vi "Edit a Button--Material.vi"() -> ()   [LabVIEW 2021, in "TSC Button Editor.lvclass"]
doc: "Edit/create buttons based on a few built-in templates.\n\n<b>Code Developed By:</b>\nTechnology Service Corporation\nwww.tsc.com/atcs\n\nDeveloper:\nDaniel Coons"
uses:
  _button-editor/TSC Button Editor.lvclass
  _button-editor/TSC Button Editor.lvclass/TSC Button Editor.ctl
  <vilib>/Utility/miscctls.llb/LVPositionTypeDef.ctl
  _button-editor/Image List Column--constant.vi
  _button-editor/Button Editor Config--constant.vi
  controls/subpanel--button preview.vi
  <vilib>/Utility/libraryn.llb/Get File Extension.vi
  <vilib>/Utility/colorconv.llb/RGB to Color.vi
  <vilib>/Utility/file.llb/Dflt Data Dir.vi
  <vilib>/Utility/libraryn.llb/Check if File or Folder Exists.vi
  <vilib>/Utility/libraryn.llb/Create Directory Recursive.vi
  user32.dll
  Material Theme/Material Theme.lvclass
  Material-Scheme/Material-Scheme.lvclass
panel:
  in  "Save For:":string(combo)
  in  "Tab Control 2":enum32{"Button Format", "Glyphs"}(tab)
  in  "Lock Text in Center?":bool
  in  "update text format":bool
  in  "Boolean Colors":T1={"false color"={"border"=15922170, "fill"=15922170}, "true color"={"border"=14936305, "fill"=14936305}, "click false color"={"border"=14410221, "fill"=14410221}, "click true color"={"border"=14410221, "fill"=14410221}, "hover false color"={"border"=14540516, "fill"=14540516}, "hover true color"={"border"=14540516, "fill"=14540516}}
  in  "Boolean Text Format":T2={"Font:Color"=3563918, "Font:Bold?"=TRUE, "Font:Name"="App Font", "Font:Size"=22}
  in  "Boolean Text":string
  in  "update colors":bool
  in  "Button Size":cluster{"Width":u32, "Height":u32}={"Width"=204, "Height"=48}
  in  "update button size":bool
  in  "Button Text Location":cluster{"Left":i32, "Top":i32}
  in  "update button text location":bool
  in  "edit":bool
  out "Images":T3(array[cluster]) caption="Array"
  in  "Filter":string
  out "images directory":path
  in  "Button Family":u16(ring) items=["(1) Small Button Single Image 24px", "(2) Small Button Text Only", "(3) Large Button Single Image 40px", "(4) Large Button Text Only", "(5) Small Button Multi Image 24px", "(6) Large Button Multi Image 40px", "(7) Floating Action Button (FAB)"]
  in  "Color Level":u16(ring) items=["Primary", "Secondary", "Tertiary", "Error", "Primary Fixed", "Secondary Fixed", "Tertiary Fixed"]
  in  "Theme":u16(ring) items=["Light Theme", "Light Medium Contrast", "Light High Contrast", "Dark Theme", "Dark Medium Contrast", "Dark High Constrast"]
  in  "theme path":path
  in  "Open":bool
  in  "Button Type":u16(ring) items=["elevated--rectangular--icon.ctl", "elevated--rounded--icon.ctl", "filled--rectangular--icon.ctl", "filled--rounded--icon.ctl", "nooutline--rectangular--icon.ctl", "nooutline--rounded--icon.ctl", "outline--rectangular--icon.ctl", "outline--rounded--icon.ctl", "tonal--rectangular--icon.ctl", "tonal--rounded--icon.ctl", "transparent--rectangular--icon.ctl", "transparent--rounded--icon.ctl"]
  in  "Tab Control":enum32{"Button Formatting"}(tab)
  in  "Image Color":u32(colorbox)=3563918
  in  "Button Image":path
  in  "Button Images":T4
  in  "Multiple Colors":T5={"False Color"=3563918, "True Color"=3563918, "True Press"=3563918, "False Press"=3563918}
  out "b":u8
  out "g":u8
  out "r":u8
  out "Color":u32(colorbox)
  in  "Hex Color":u32 max=16777215 format="%06x"
  in  "close":bool
  out "header":bool
  in  "Save":bool
  out "error out":errorcluster
  # "Download a folder of icons here: https://github.com/danielcoons/material-icons-toolkit<Material-Toolkit> to easily sort by size and connect to directory"
  # "drag and drop on glyph Button Image path control to add"
  # "Note: match the size of the replacement image so scaling is correct.\nNormal size: 24x24px, Large size: 40x40px, Icon size: 30x30px\n\nFor other desired sizes, save the control and open it in LabVIEW. Use the edit mode features to replace the picture items. Making sure the image doesn't try to resize is important for it to look correct."
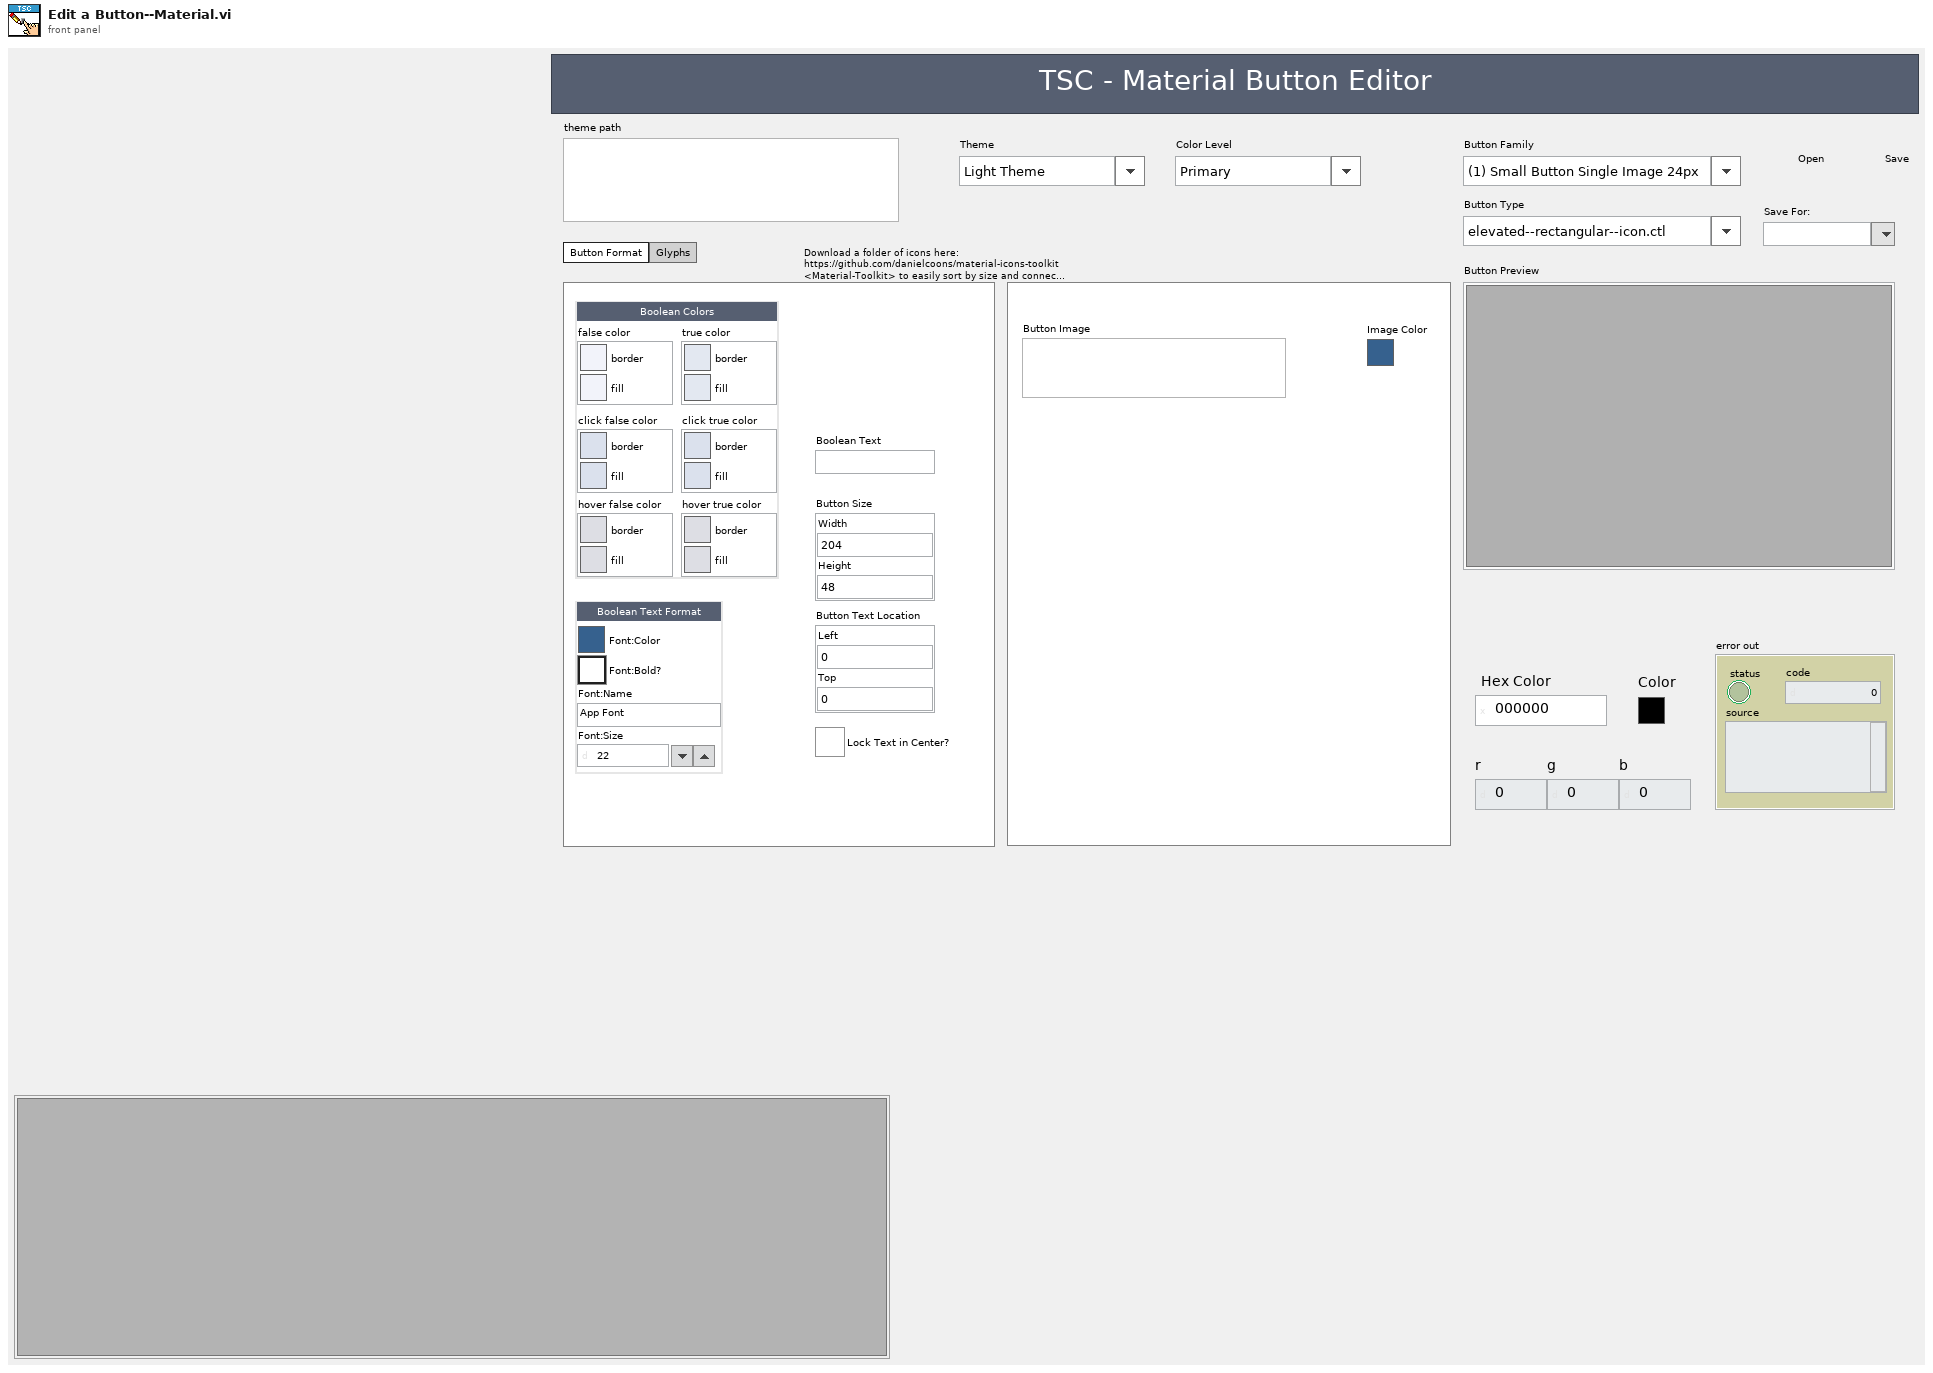
[diagram p1: front panel]
types:
  T1 = cluster{"false color":cluster{"border":u32, "fill":u32}, "true color":cluster{"border":u32, "fill":u32}, "click false color":cluster{"border":u32, "fill":u32}, "click true color":cluster{"border":u32, "fill":u32}, "hover false color":cluster{"border":u32, "fill":u32}, "hover true color":cluster{"border":u32, "fill":u32}}
  T2 = cluster{"Font:Color":u32, "Font:Bold?":bool, "Font:Name":string, "Font:Size":u32}
  T3 = cluster{"2D Picture":picture, "path":path, "image-name":string}[][]
  T4 = cluster{"False Image":path, "True Image":path, "True Press":path, "False Press":path}
  T5 = cluster{"False Color":u32, "True Color":u32, "True Press":u32, "False Press":u32}
  T6 = cluster{"2D Picture":picture, "path":path, "image-name":string}[]
  T7 = typedef "TSC Button Editor.lvclass/User Events--typedef.ctl" = cluster{"update colors":refnum<user-event>, "update boolean data":refnum<user-event>, "update image":refnum<user-event>, "update multi image":refnum<user-event>}
  T8 = typedef "LVPositionTypeDef.ctl" = cluster{"Left":i32, "Top":i32}
  T9 = enum32{"invalid VI type", "Standard VI", "Control VI", "Global VI", "Polymorphic VI", "Configuration VI", "SubSystem", "Facade VI", "Method VI", "Statechart Diagram VI"}
  T10 = typedef "LVBoundsTypeDef.ctl" = cluster{"Width":u32, "Height":u32}
  T11 = cluster{"2D Picture":picture, "path":path, "image-name":string}
  T12 = typedef "LVPoint32TypeDef.ctl" = cluster{"Horizontal":i32, "Vertical":i32}
  T13 = cluster{"data name":string, "drag data":variant}[]
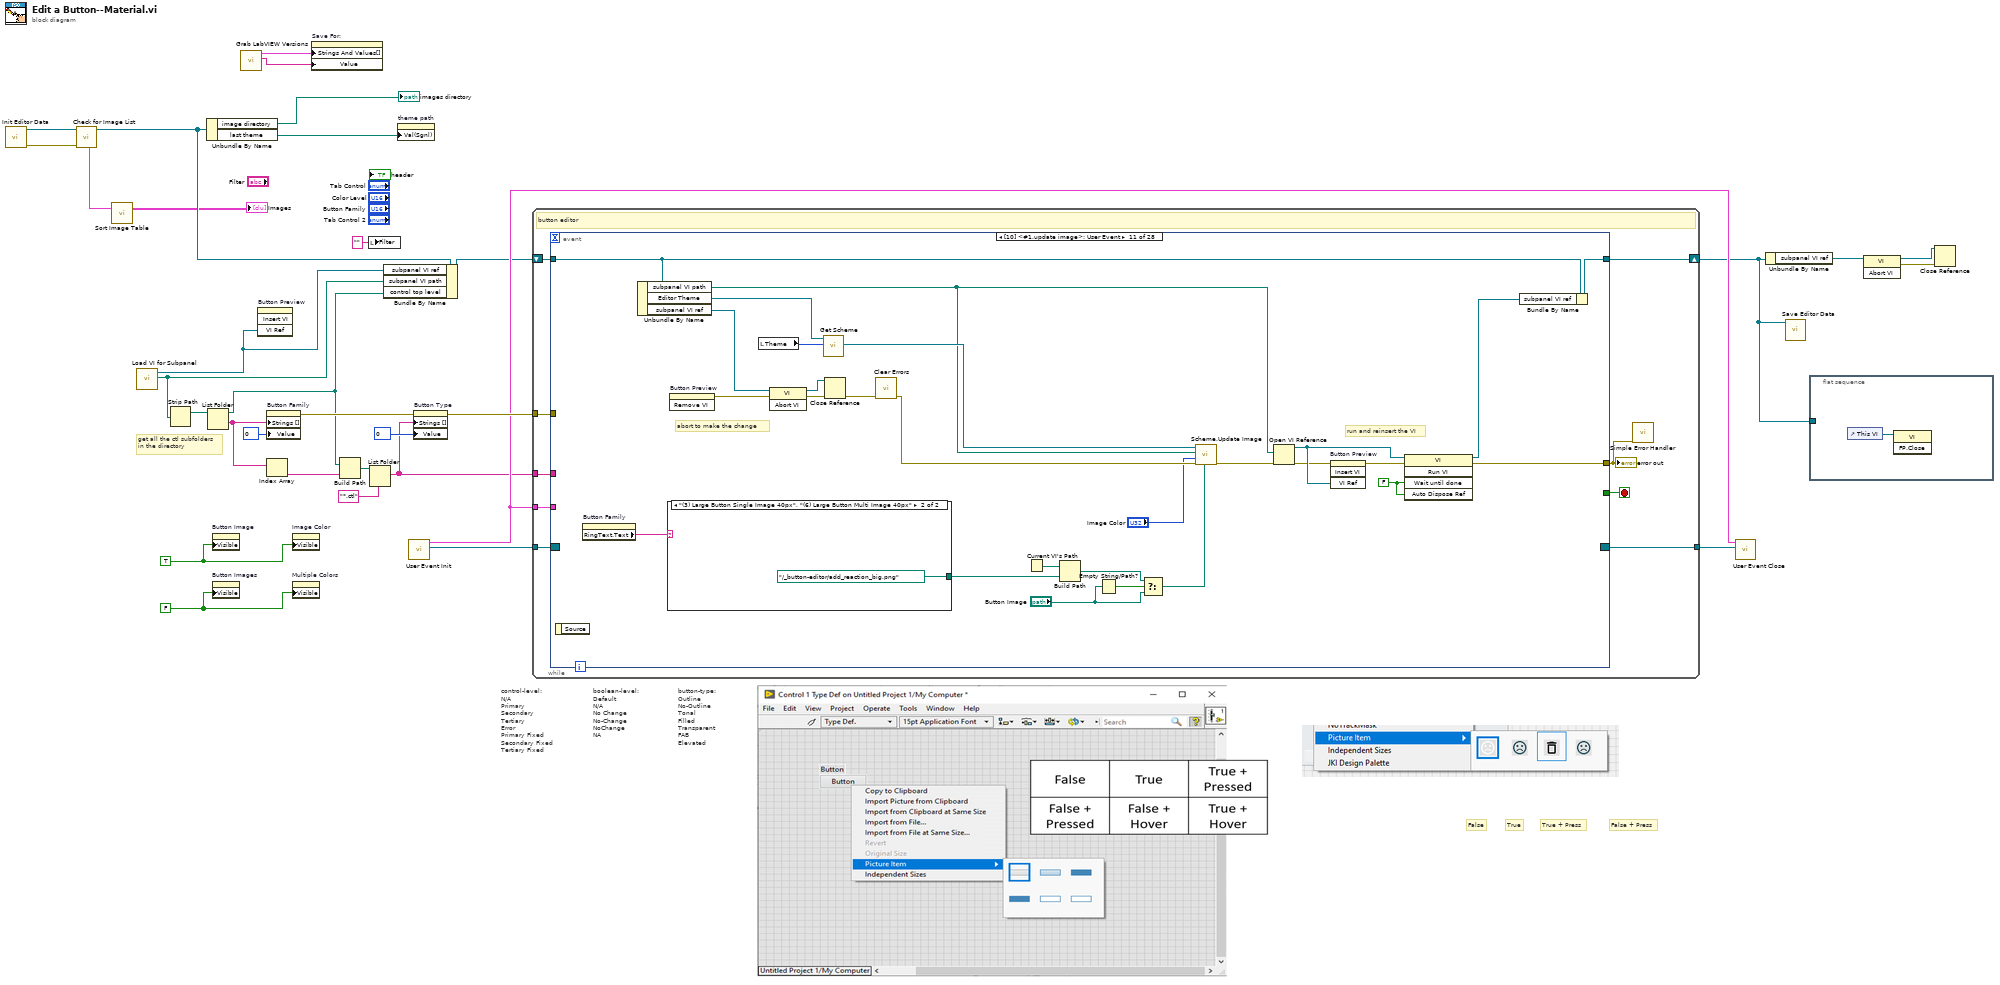
[diagram p0: block diagram]
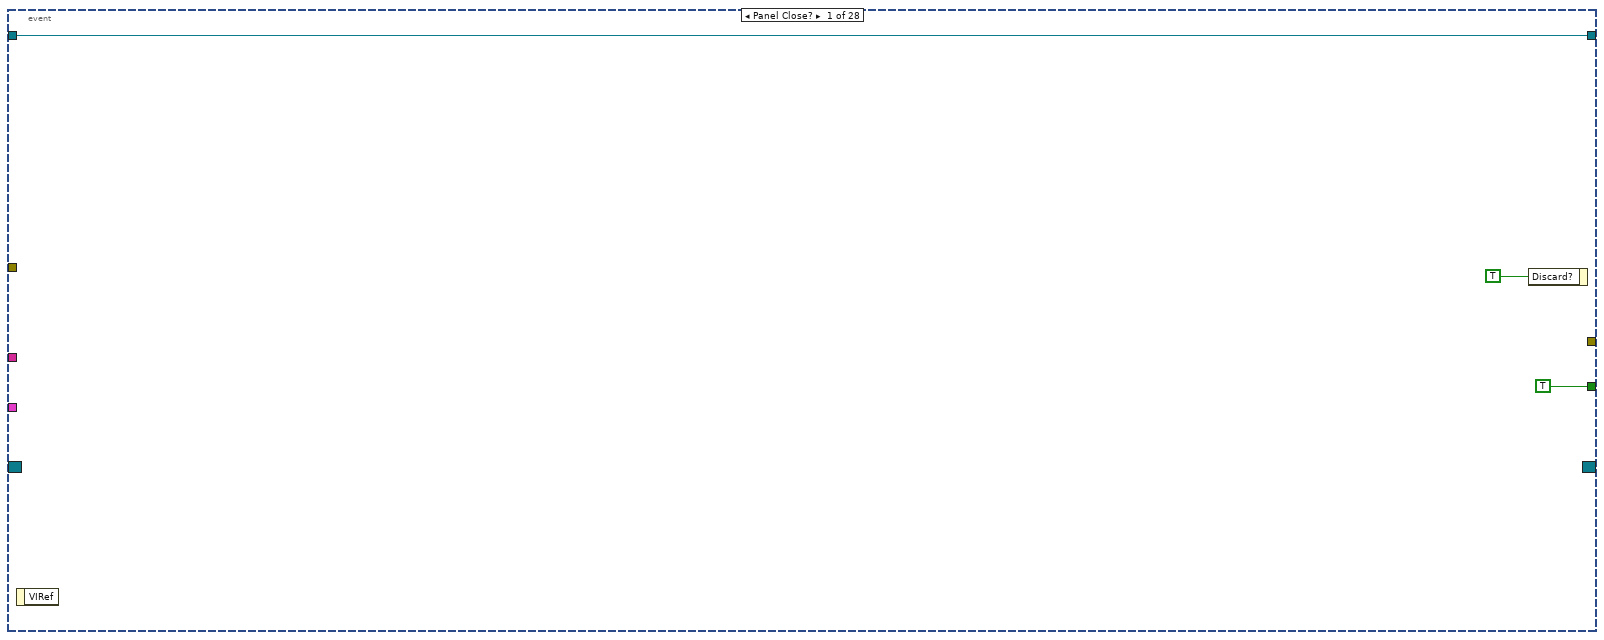
[diagram p2: hidden frame]
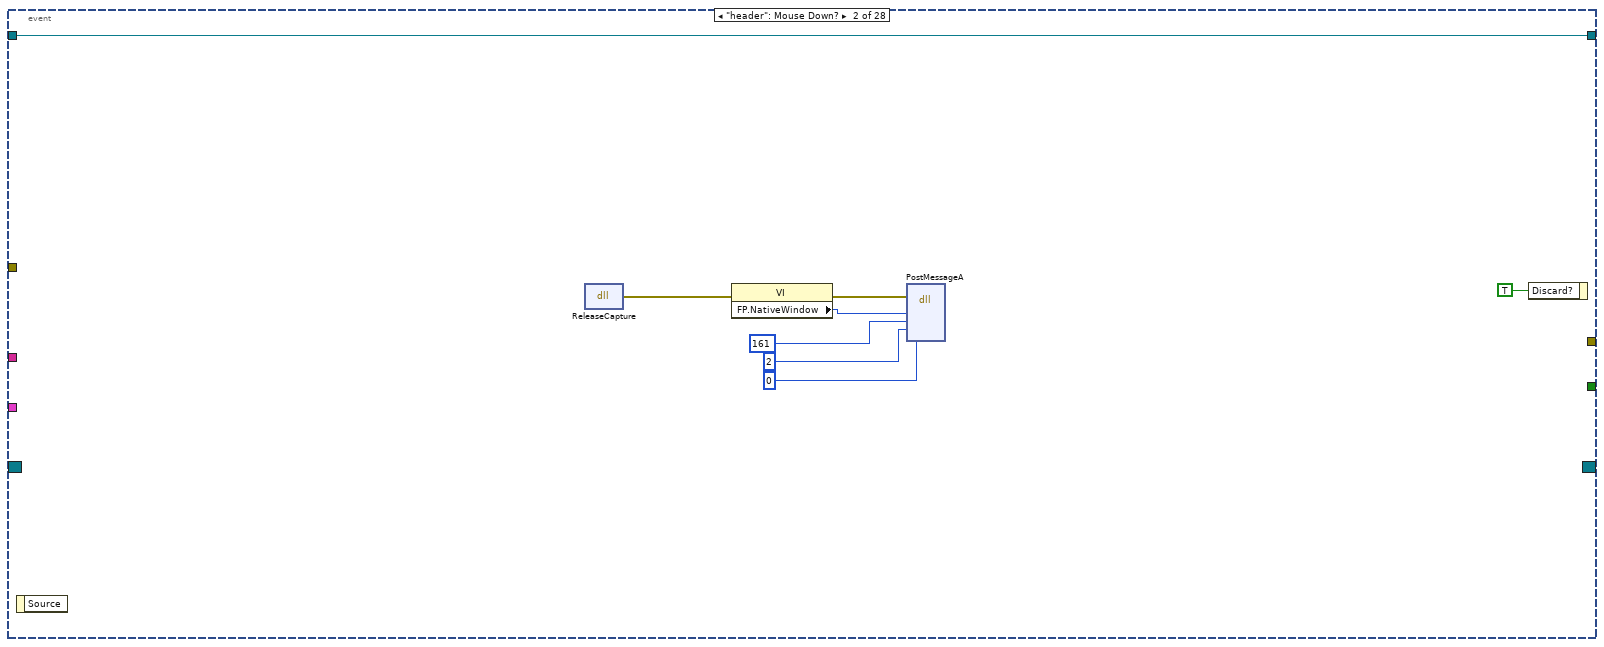
[diagram p3: hidden frame]
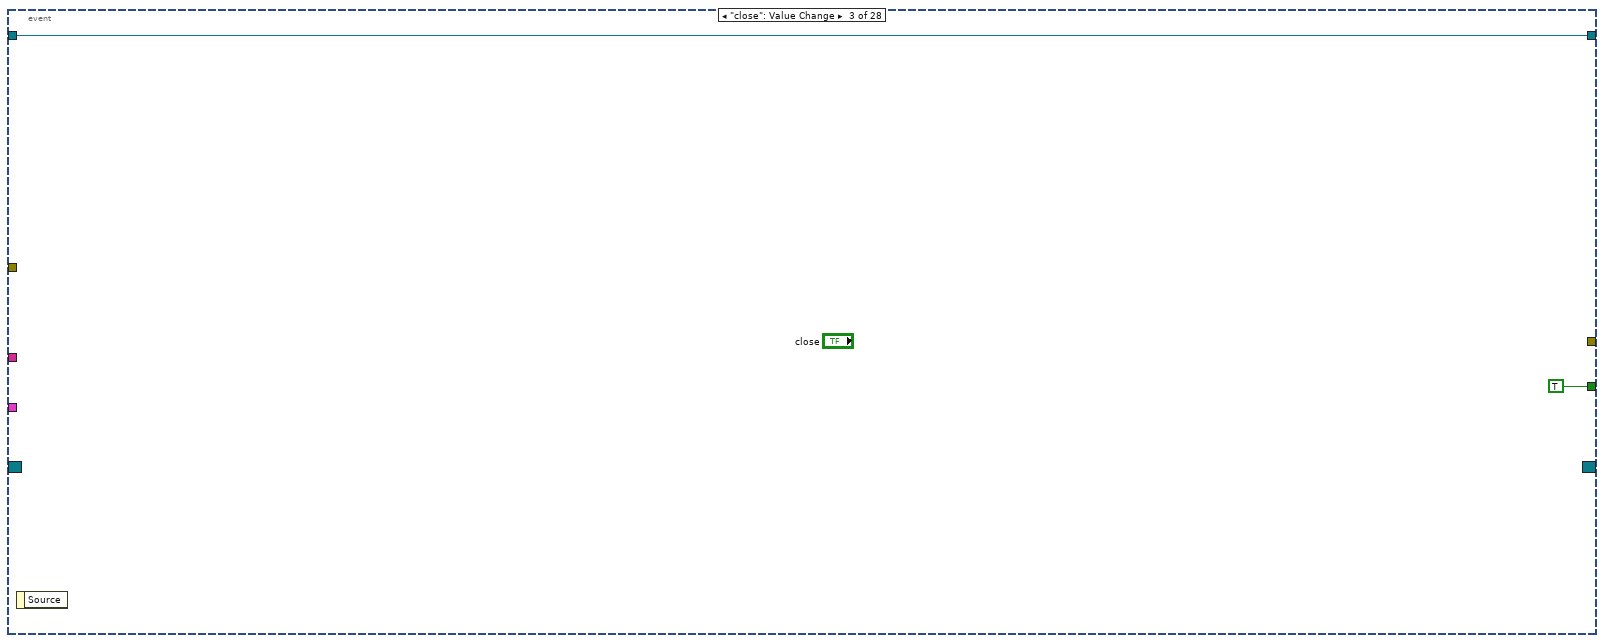
[diagram p4: hidden frame]
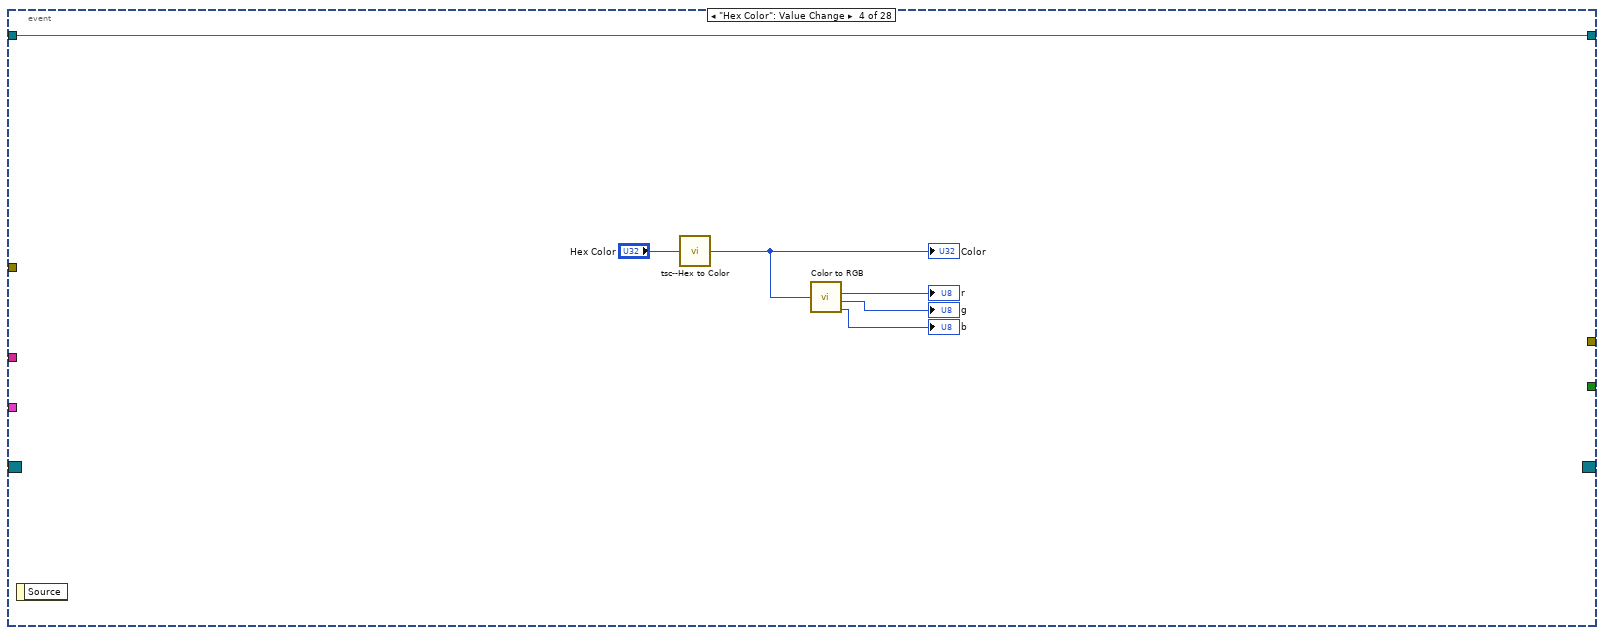
[diagram p5: hidden frame]
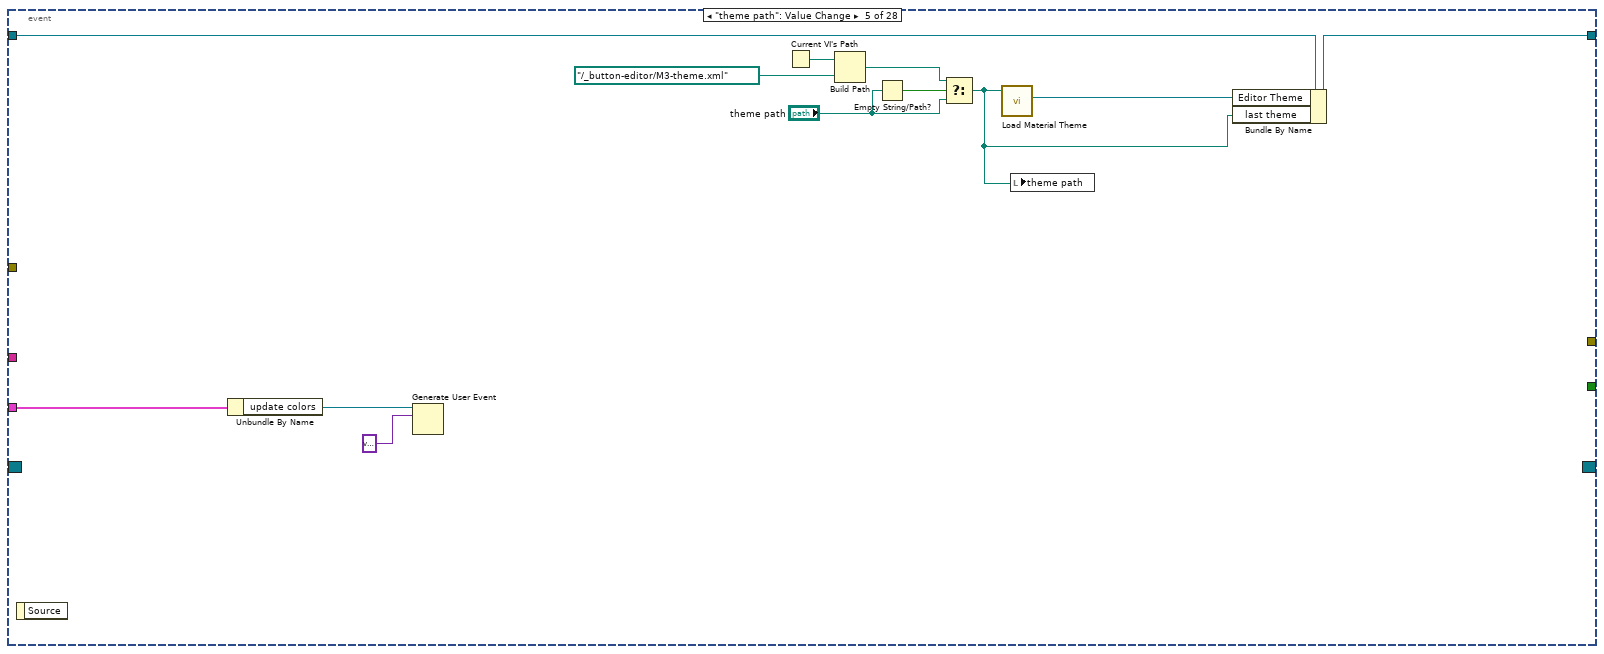
[diagram p6: hidden frame]
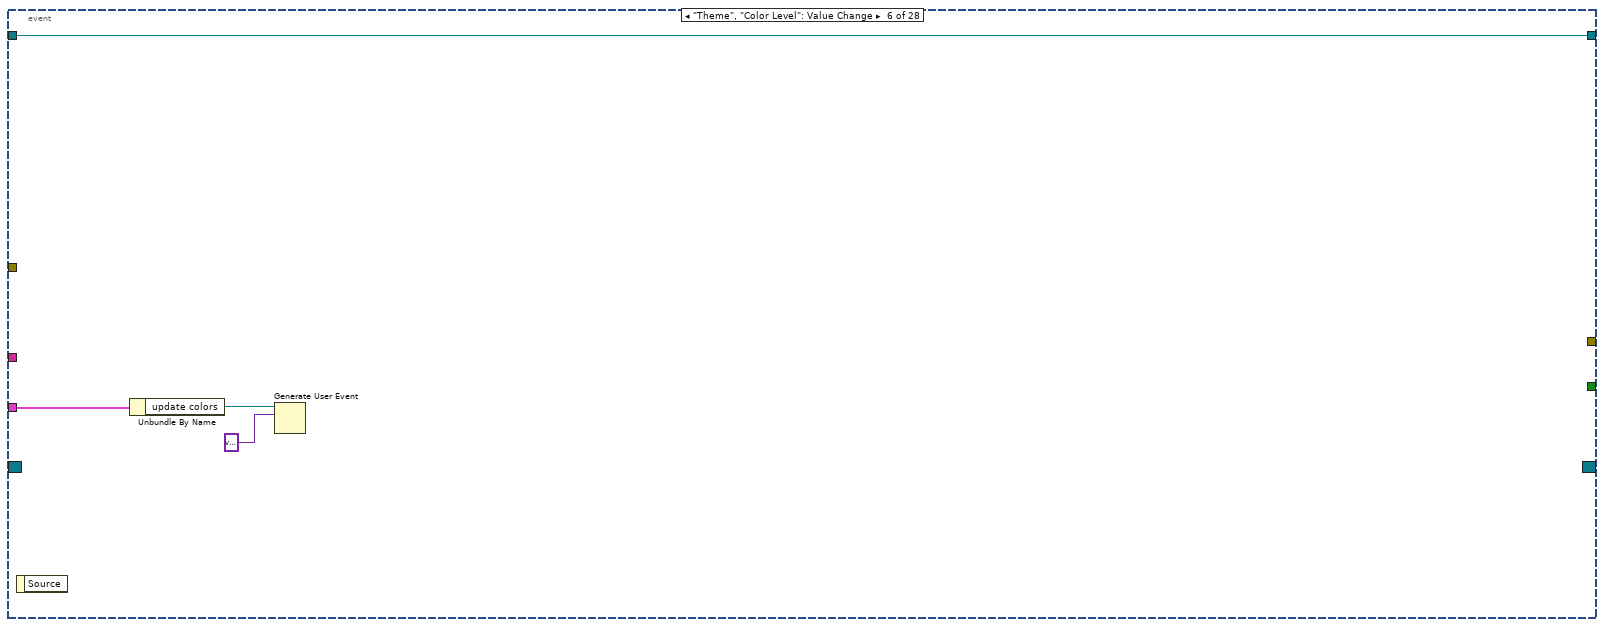
[diagram p7: hidden frame]
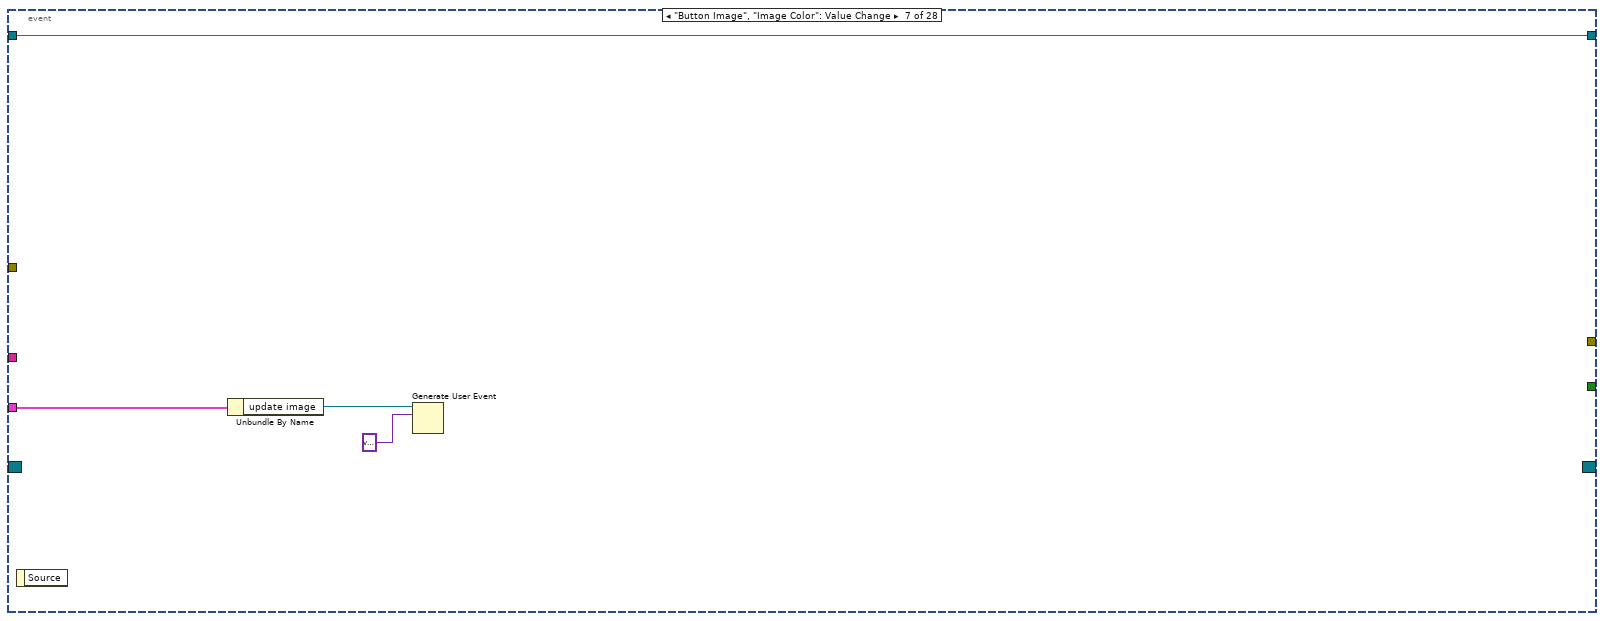
[diagram p8: hidden frame]
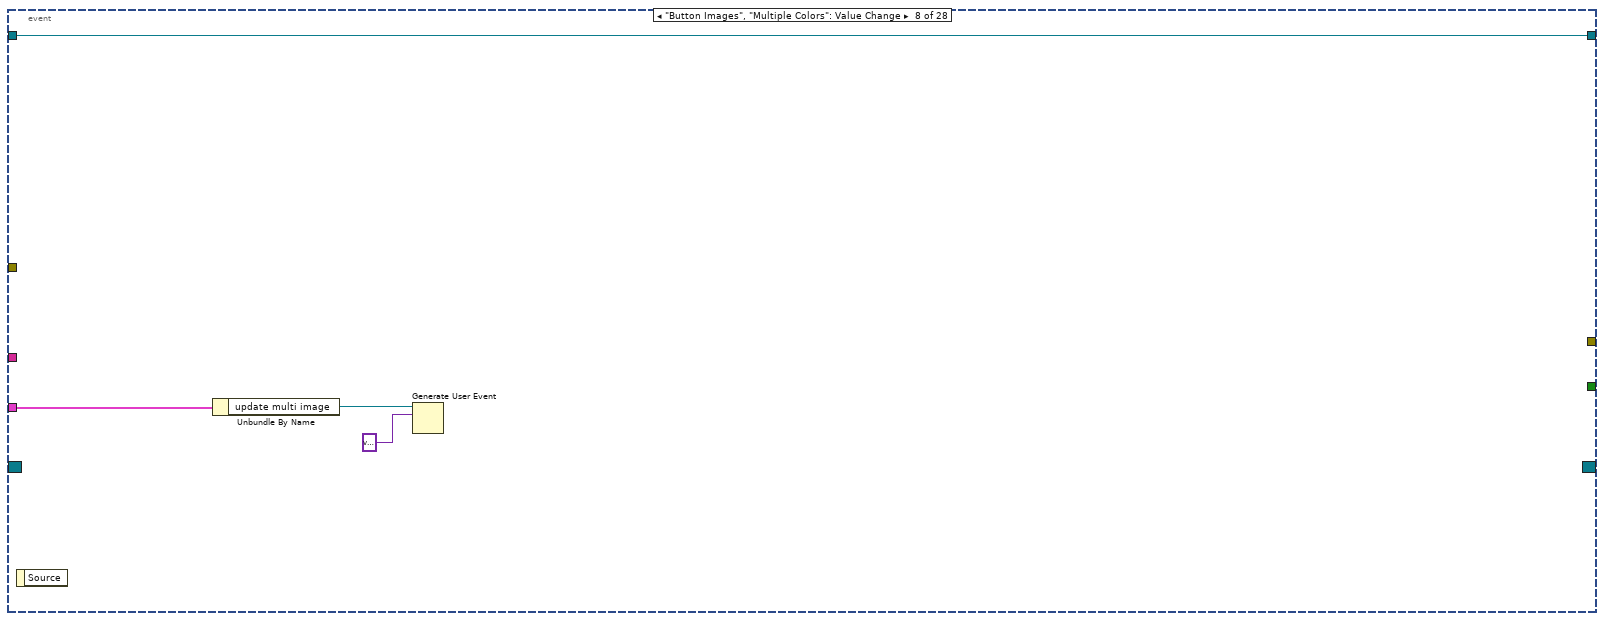
[diagram p9: hidden frame]
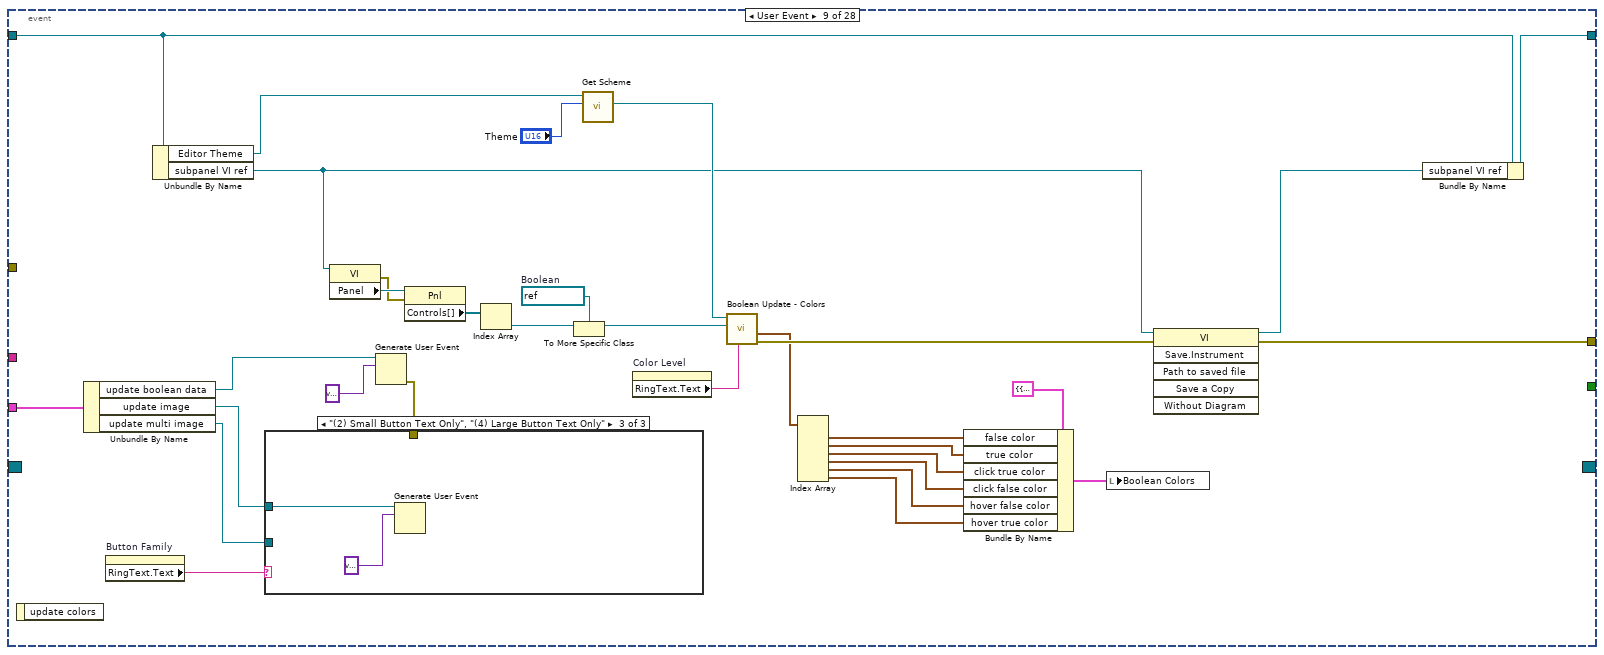
[diagram p10: hidden frame]
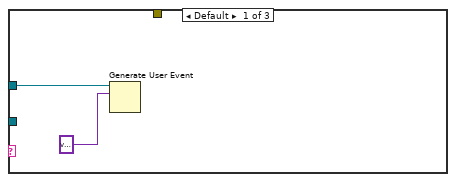
[diagram p11: hidden frame]
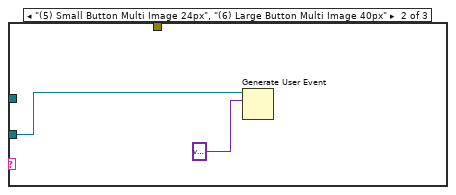
[diagram p12: hidden frame]
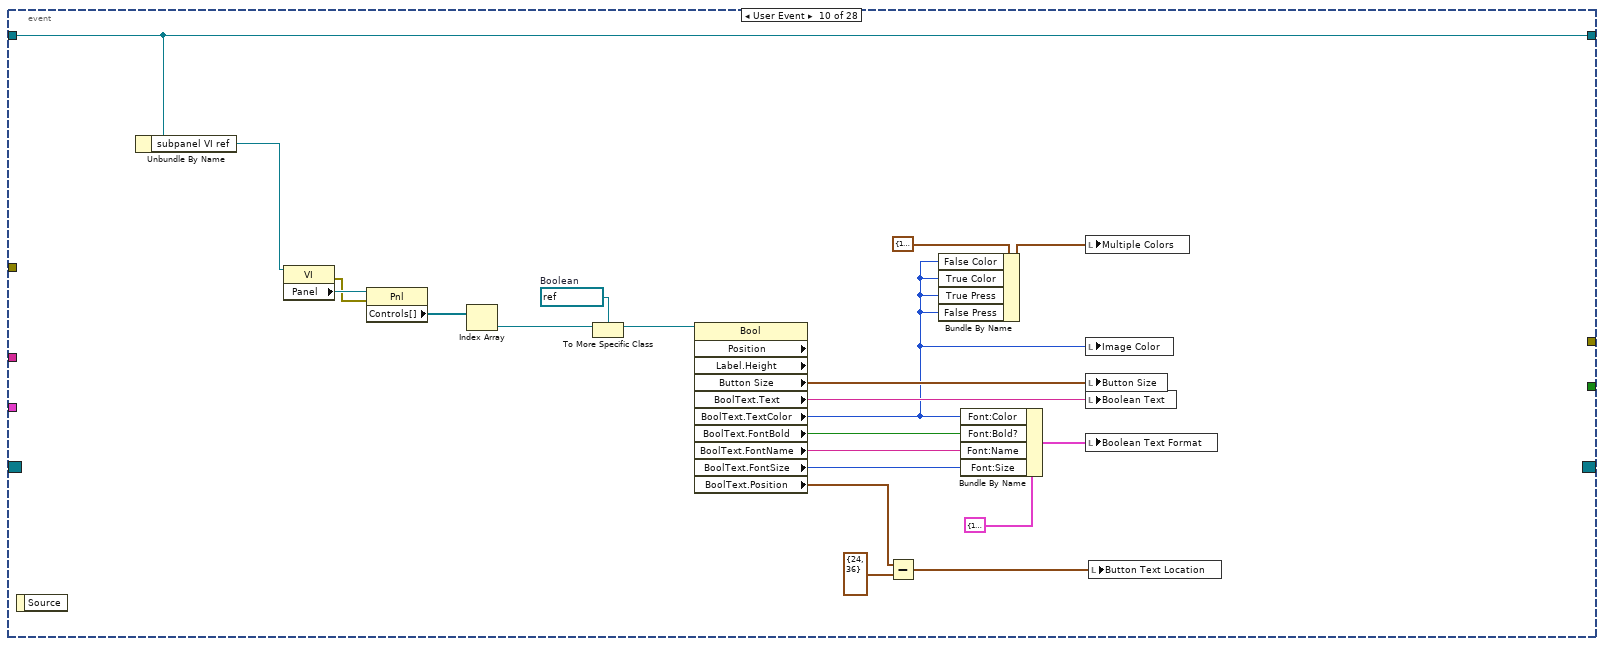
[diagram p13: hidden frame]
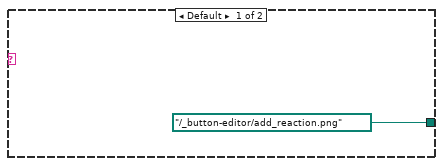
[diagram p14: hidden frame]
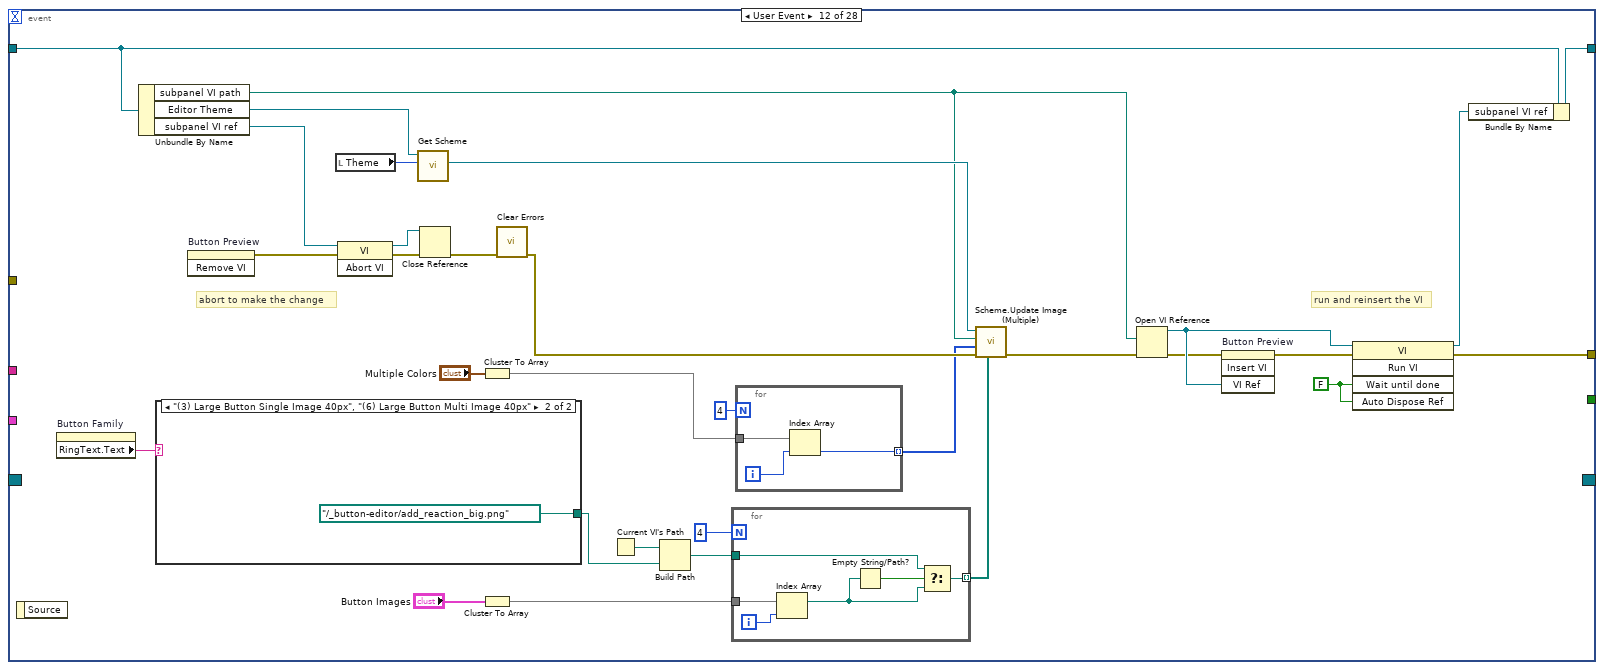
[diagram p15: hidden frame]
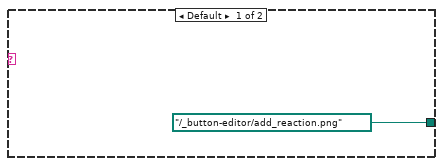
[diagram p16: hidden frame]
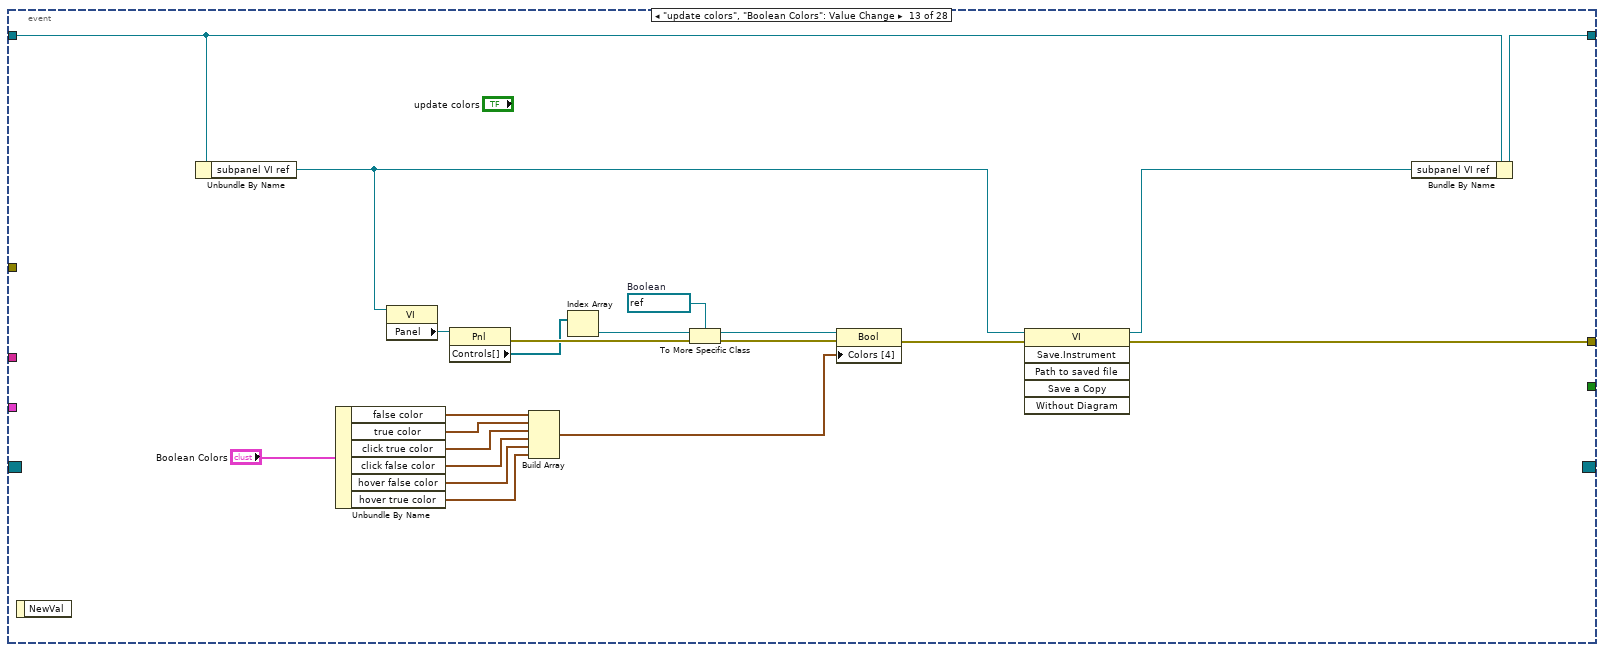
[diagram p17: hidden frame]
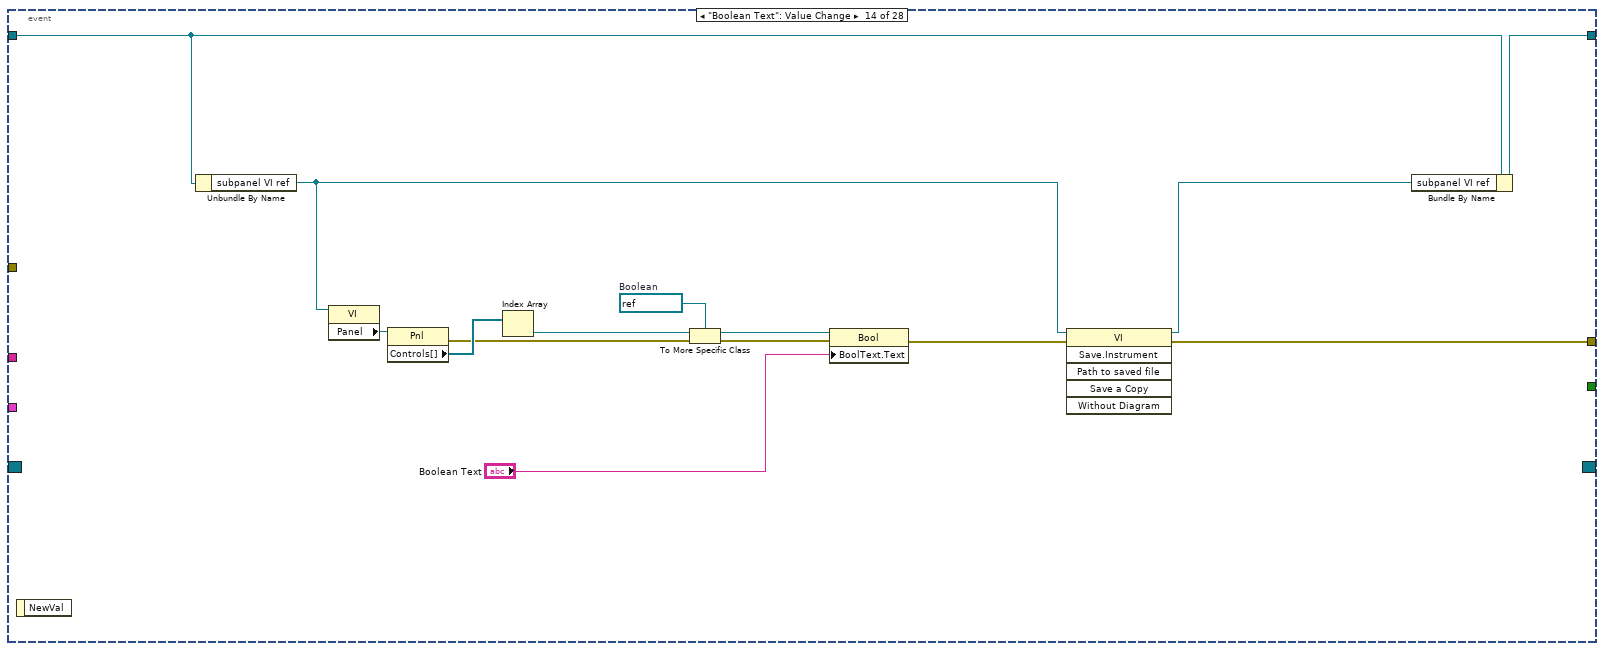
[diagram p18: hidden frame]
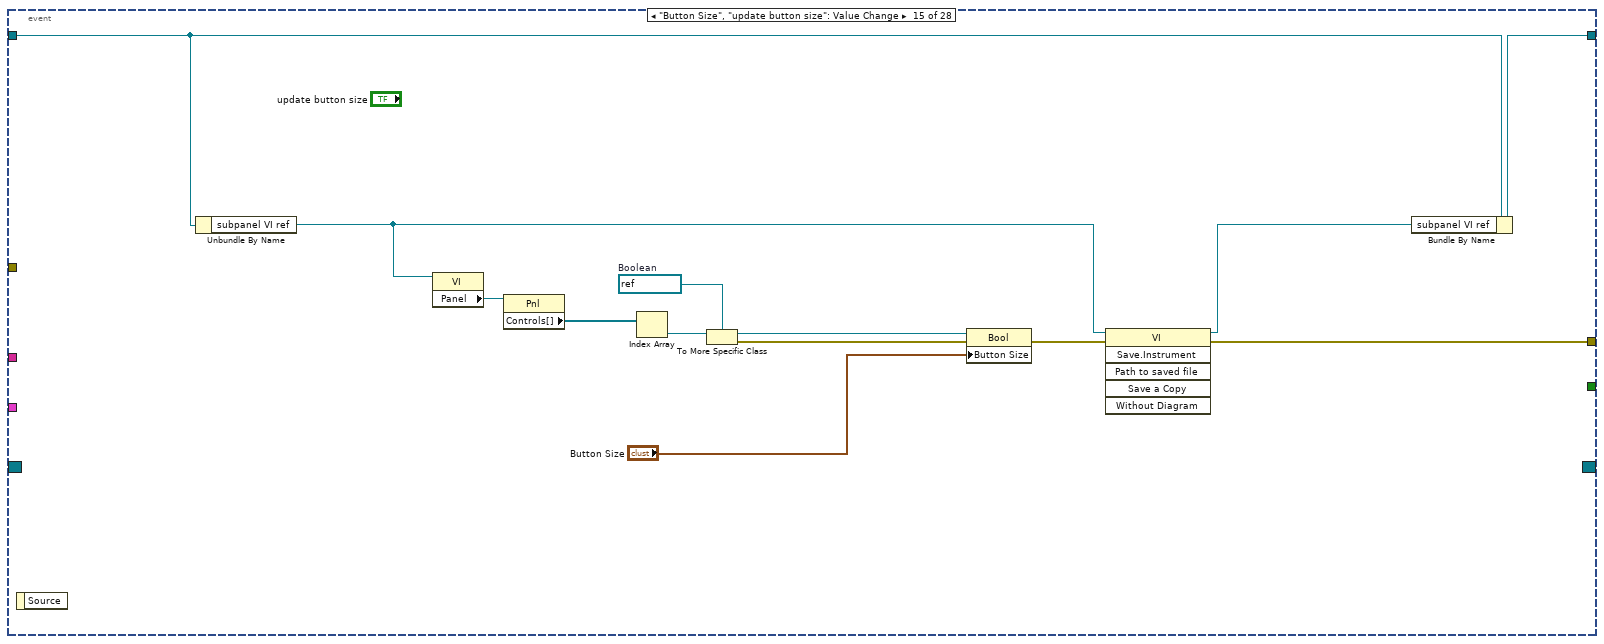
[diagram p19: hidden frame]
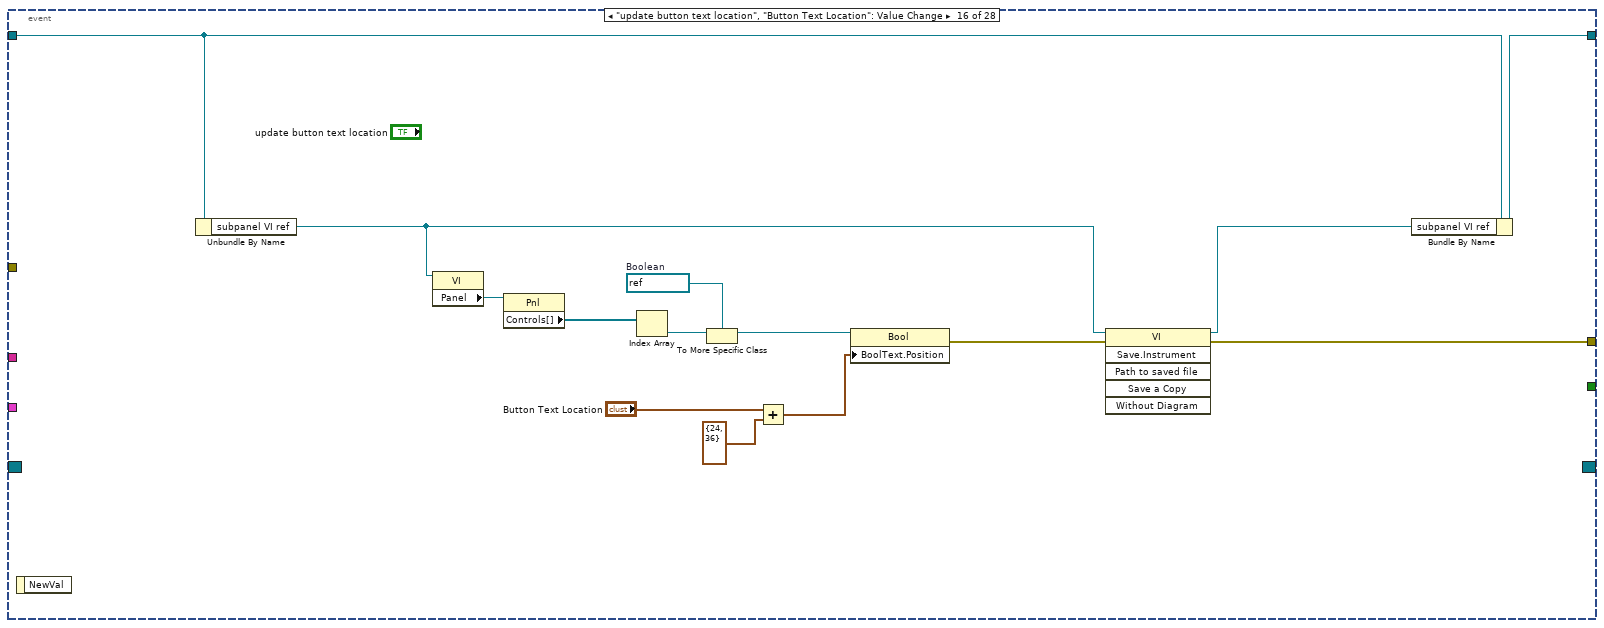
[diagram p20: hidden frame]
diagram:
  w17 = FALSE
  w18 = TRUE
  w20 = u16 0 items=[""] ("Button Type")
  w25 = u16 0 items=[""] ("Button Family")
  # "button-type:\nOutline\nNo-Outline\nTonal\nFilled\nTransparent\nFAB\nElevated"
  # "boolean-level:\nDefault\nN/A\nNo Change\nNo-Change\nNoChange\nNA"
  # "control-level:\nN/A\nPrimary\nSecondary\nTertiary\nError\nPrimary Fixed\nSecondary Fixed\nTertiary Fixed"
  # "False + Press"
  # "True + Press"
  # "True"
  # "False"
  # "get all the ctl subfolders\nin the directory"
  n1 = call "Init Editor Data.vi"() -> ("error out"=w6:errorcluster, "TSC Button Editor"=w10:refnum<class "TSC Button Editor.lvclass">)  [unwired: 10 in]
  n2 = call "Check for Image List.vi"("error in"=w6, "TSC Button Editor in"=w10) -> ("TSC Button Editor out"=w9:refnum<class "TSC Button Editor.lvclass">, "Images"=w8:T6)  [unwired: 7 in, 1 out]
  n3 = call "Sort Image Table.vi"("Images in"=w8) -> ("Images out"=→"Images":T3)  [unwired: 2 in]
  n4 = call "Load VI for Subpanel.vi"() -> ("VI Path"=w12:path, "VI out"=w13:refnum<vi>)  [unwired: 10 in]
  n5 = Strip Path(path=w12) -> (stripped path=w30:path)  [unwired: 1 out]
  n6 = Unbundle By Name(w9) -> ("image directory"=→"images directory":path, "last theme"=w16:path)
  n7 = List Folder(path=w30) -> (path out=w5:path, folder names=w24:string[])  [unwired: 3 in, 2 out]
  n8 = property on="Button Image" class="Path"("Visible"=w18) -> ()  [unwired: 2 in, 2 out]
  n9 = property on="Button Images" class="Clust (strict)"("Visible"=w17) -> ()  [unwired: 2 in, 2 out]
  n10 = call "Grab LabVIEW Versions.vi"() -> ("Selection"=w1:string, "Strings and Values"=w2:cluster{"string":string, "value":string}[])  [unwired: 10 in]
  n11 = invoke on="Button Preview" class="SubPnl" method="Insert VI"("VI Ref"=w13) -> ()  [unwired: 3 in, 4 out]
  n12 = property on="Button Family" class="Ring (strict)"("Strings []"=w24, "Value"=w25) -> (error out=w26:errorcluster)  [unwired: 2 in, 1 out]
  n13 = Index Array(array=w24) -> (element=w23:string)  [unwired: 1 in]
  n14 = property on="Image Color" class="ColBox"("Visible"=w18) -> ()  [unwired: 2 in, 2 out]
  n15 = property on="Multiple Colors" class="Clust (strict)"("Visible"=w17) -> ()  [unwired: 2 in, 2 out]
  n16 = property on="Save For:" class="CmbBox"("Strings And Values[]"=w2, "Value"=w1) -> ()  [unwired: 2 in, 2 out]
  n17 = Build Path(base path=w5, name or relative path=w23) -> (appended path=w22:path)
  n18 = local write "Filter"("" ("Filter")) -> ()
  n19 = List Folder(path=w22, pattern="*.ctl") -> (filenames=w19:string[])  [unwired: 2 in, 3 out]
  n20 = Bundle By Name(cluster=w9, "subpanel VI ref"=w13, "subpanel VI path"=w12, "control top level"=w5) -> (w14:refnum<class "TSC Button Editor.lvclass">)
  n21 = property on="theme path" class="Path"("Val(Sgnl)"=w16) -> ()  [unwired: 2 in, 2 out]
  n22 = call "User Event Init.vi"() -> ("Event Registration Refnum"=w29:refnum<event-registration>, "user events"=w27:T7)  [unwired: 10 in]
  n23 = property on="Button Type" class="Ring (strict)"(error in=w26, "Strings []"=w19, "Value"=w20) -> (error out=w31:errorcluster)  [unwired: 1 in, 1 out]
  n24 = while {
    tunnel: w31 -> [w41]
    tunnel: w29 -> [w40]
    tunnel: [w39] -> w28
    tunnel: w27 -> [w38]
    tunnel: w19 -> [w37]
    shift-right: [w34] -> w3
    shift-left: w14 -> [w35]
    stop <- w42 stop-if-true
    # "button editor"
    n25 = event shown="[10] <#1.update image>: User Event" {
      selector: w40 -> [_ _ _ _ _ _ _ _ _ _ _ _ _ _ _ _ _ _ _ _ _ _ _ _ _ _ _ _]
      dyn-events: [_ _ _ _ _ _ _ _ _ _ _ _ _ _ _ _ _ _ _ _ _ _ _ _ _ _ _ _] -> w39
      timeout: _ -> [_ _ _ _ _ _ _ _ _ _ _ _ _ _ _ _ _ _ _ _ _ _ _ _ _ _ _ _]
      tunnel: [TRUE _ TRUE _ _ _ _ _ _ _ _ _ _ _ _ _ _ _ _ _ _ _ _ _ _ _ _ _] -> w42
      tunnel: [_ _ _ _ _ _ _ _ w112 _ w158 w192 w233 w245 w255 w264 w281 w296 w317 w345 w401 _ w431 w522 _ _ _ _] -> w36
      tunnel: w41 -> [_ _ _ _ _ _ _ _ _ _ _ _ _ _ _ _ _ _ _ _ _ _ _ _ _ _ _ _]
      tunnel: w38 -> [_ _ _ _ w73 w77 w81 w85 w113 _ _ _ _ _ _ _ _ _ _ _ w390 _ _ _ _ _ _ _]
      tunnel: w37 -> [_ _ _ _ _ _ _ _ _ _ _ _ _ _ _ _ _ _ _ _ _ _ _ _ _ _ _ _]
      tunnel: w35 -> [w43 w46 w54 w56 w65 w74 w78 w82 w90 w125 w147 w176 w219 w238 w252 w267 w279 w294 w313 w343 w380 w414 w429 w521 w543 w579 w590 w597]
      tunnel: [w43 w46 w54 w56 w64 w74 w78 w82 w88 w125 w146 w175 w218 w237 w251 w266 w280 w295 w313 w343 w379 w414 w428 w519 w540 w579 w590 w597] -> w34
      event Panel Close? {
        n26 = event-data() -> ()  [unwired: 1 in, 1 out]
        n27 = event-data("Discard?"=TRUE) -> ()  [unwired: 1 in, 1 out]
      }
      event "header": Mouse Down? {
        n28 = event-data() -> ()  [unwired: 1 in, 1 out]
        n29 = dll-call lib="user32.dll" fn="ReleaseCapture"() -> (error out=w49:errorcluster)  [unwired: 4 in, 1 out]
        n30 = property class="VI"(error in=w49) -> (error out=w48:errorcluster, "FP.NativeWindow"=w47:u64)  [unwired: 1 in, 1 out]
        n31 = dll-call lib="user32.dll" fn="PostMessageA"(error in=w48, "hWnd"=w47, "Msg"=161, "wParam"=2, "lParam"=0) -> ()  [unwired: 7 in, 2 out]
        n32 = event-data("Discard?"=TRUE) -> ()  [unwired: 1 in, 1 out]
      }
      event "close": Value Change {
        n33 = event-data() -> ()  [unwired: 1 in, 1 out]
      }
      event "Hex Color": Value Change {
        n34 = event-data() -> ()  [unwired: 1 in, 1 out]
        n35 = call "tsc--Hex to Color.vi"("Hex String"="Hex Color") -> ("Color"=w57:u32)  [unwired: 4 in]
        "Color" <- w57
        n36 = call <vilib>:"Color to RGB.vi"("Color"=w57) -> ("R"=→"r":u8, "G"=→"g":u8, "B"=→"b":u8)  [unwired: 1 out]
      }
      event "theme path": Value Change {
        n37 = event-data() -> ()  [unwired: 1 in, 1 out]
        n38 = Unbundle By Name(w73) -> ("update colors"=w71:refnum<user-event>)
        n39 = Generate User Event(user event=w71, event data cluster=variant ("event data")) -> ()  [unwired: 2 in, 2 out]
        n40 = Current VI's Path() -> (path=w69:path)
        n41 = Build Path(base path=w69, name or relative path=path "../_button-editor/M3-theme.xml") -> (appended path=w67:path)
        n42 = Empty String/Path?(string/path="theme path") -> (empty?=w70:bool)
        n43 = Select(t=w67, s=w70, f="theme path") -> (s? t:f=w62:path)
        n44 = call "Load Material Theme.vi"("file path (use dialog)"=w62) -> ("Theme"=w63:refnum<class "Material Theme.lvclass">)  [unwired: 9 in, 1 out]
        n45 = local write "theme path"(w62) -> ()
        n46 = Bundle By Name(cluster=w65, "Editor Theme"=w63, "last theme"=w62) -> (w64:refnum<class "TSC Button Editor.lvclass">)
      }
      event "Theme", "Color Level": Value Change {
        n47 = event-data() -> ()  [unwired: 1 in, 1 out]
        n48 = Unbundle By Name(w77) -> ("update colors"=w75:refnum<user-event>)
        n49 = Generate User Event(user event=w75, event data cluster=variant ("event data")) -> ()  [unwired: 2 in, 2 out]
      }
      event "Button Image", "Image Color": Value Change {
        n50 = event-data() -> ()  [unwired: 1 in, 1 out]
        n51 = Unbundle By Name(w81) -> ("update image"=w79:refnum<user-event>)
        n52 = Generate User Event(user event=w79, event data cluster=variant ("event data")) -> ()  [unwired: 2 in, 2 out]
      }
      event "Button Images", "Multiple Colors": Value Change {
        n53 = event-data() -> ()  [unwired: 1 in, 1 out]
        n54 = Unbundle By Name(w85) -> ("update multi image"=w83:refnum<user-event>)
        n55 = Generate User Event(user event=w83, event data cluster=variant ("event data")) -> ()  [unwired: 2 in, 2 out]
      }
      event User Event {
        w102 = refnum<vi> refnum  # Boolean
        n56 = event-data() -> ()  [unwired: 1 in, 1 out]
        n57 = Unbundle By Name(w113) -> ("update boolean data"=w115:refnum<user-event>, "update image"=w109:refnum<user-event>, "update multi image"=w110:refnum<user-event>)
        n58 = property on="Button Family" class="Ring (strict)"() -> ("RingText.Text"=w111:string)  [unwired: 2 in, 2 out]
        n59 = Unbundle By Name(w90) -> ("Editor Theme"=w86:refnum<class "Material Theme.lvclass">, "subpanel VI ref"=w89:refnum<vi>)
        n60 = property class="VI"(reference=w89) -> (error out=w104:errorcluster, "Panel"=w107:refnum<vi>)  [unwired: 1 in, 1 out]
        n61 = Generate User Event(user event=w115, event data cluster=variant ("event data")) -> (error out=w108:errorcluster)  [unwired: 2 in, 1 out]
        n62 = case shown="\"(2) Small Button Text Only\", \"(4) Large Button Text Only\"" w111 {
          tunnel: w110 -> [_ w120 _]
          tunnel: w109 -> [w118 _ w122]
          tunnel: w108 -> [_ _ _]
          frame Default {
            n63 = Generate User Event(user event=w118, event data cluster=variant ("event data")) -> ()  [unwired: 2 in, 2 out]
          }
          frame "(5) Small Button Multi Image 24px", "(6) Large Button Multi Image 40px" {
            n64 = Generate User Event(user event=w120, event data cluster=variant ("event data")) -> ()  [unwired: 2 in, 2 out]
          }
          frame "(2) Small Button Text Only", "(4) Large Button Text Only" {
            n65 = Generate User Event(user event=w122, event data cluster=variant ("event data")) -> ()  [unwired: 2 in, 2 out]
          }
        }
        n66 = property class="Pnl"(reference=w107, error in=w104) -> ("Controls[]"=w106:refnum<vi>[])  [unwired: 2 out]
        n67 = Index Array(array=w106) -> (element=w105:refnum<vi>)  [unwired: 1 in]
        n68 = To More Specific Class(target class=w102, reference=w105) -> (specific class reference=w103:refnum<vi>)  [unwired: 1 in, 1 out]
        n69 = call "Get Scheme.vi"("Theme"="Theme", "Material Theme in"=w86) -> ("Material-Scheme"=w117:refnum<class "Material-Scheme.lvclass">)  [unwired: 7 in, 2 out]
        n70 = property on="Color Level" class="Ring (strict)"() -> ("RingText.Text"=w93:string)  [unwired: 2 in, 2 out]
        n71 = call "Boolean Update - Colors.vi"("control-level"=w93, "Bool Refnum"=w103, "Material-Scheme in"=w117) -> ("error out"=w101:errorcluster, "Array"=w100:cluster{"bg":u32, "fg":u32}[])  [unwired: 5 in, 2 out]
        n72 = Index Array(array=w100) -> (element #1=w98:cluster{"bg":u32, "fg":u32}, element #2=w97:cluster{"bg":u32, "fg":u32}, element #3=w91:cluster{"bg":u32, "fg":u32}, element #4=w92:cluster{"bg":u32, "fg":u32}, element #5=w96:cluster{"bg":u32, "fg":u32}, element #6=w95:cluster{"bg":u32, "fg":u32})  [unwired: 6 in]
        n73 = Bundle By Name(cluster=T1 {"false color"={"border"=15922170, "fill"=15922170}, "true color"={"border"=14936305, "fill"=14936305}, "click false color"={"border"=14410221, "fill"=14410221}, "click true color"={"border"=14410221, "fill"=14410221}, "hover false color"={"border"=14540516, "fill"=14540516}, "hover true color"={"border"=14540516, "fill"=14540516}} ("Boolean Colors"), "false color"=w98, "true color"=w97, "click true color"=w91, "click false color"=w92, "hover false color"=w96, "hover true color"=w95) -> (w94:T1)
        n74 = local write "Boolean Colors"(w94) -> ()
        n75 = invoke class="VI" method="Save.Instrument"(reference=w89, error in=w101) -> (reference out=w87:refnum<vi>, error out=w112:errorcluster)  [unwired: 4 in, 4 out]
        n76 = Bundle By Name(cluster=w90, "subpanel VI ref"=w87) -> (w88:refnum<class "TSC Button Editor.lvclass">)
      }
      event User Event {
        w140 = refnum<vi> refnum  # Boolean
        n77 = event-data() -> ()  [unwired: 1 in, 1 out]
        n78 = Unbundle By Name(w125) -> ("subpanel VI ref"=w124:refnum<vi>)
        n79 = property class="VI"(reference=w124) -> (error out=w141:errorcluster, "Panel"=w144:refnum<vi>)  [unwired: 1 in, 1 out]
        n80 = property class="Pnl"(reference=w144, error in=w141) -> ("Controls[]"=w143:refnum<vi>[])  [unwired: 2 out]
        n81 = Index Array(array=w143) -> (element=w142:refnum<vi>)  [unwired: 1 in]
        n82 = To More Specific Class(target class=w140, reference=w142) -> (specific class reference=w139:refnum<vi>)  [unwired: 1 in, 1 out]
        n83 = property class="Bool" props=["Position", "Label", "Height", "Button Size", "BoolText", "Text", "BoolText", "TextColor", "BoolText", "FontBold", "BoolText", "FontName", "BoolText", "FontSize", "BoolText", "Position"](reference=w139) -> ("Button Size"=w138:T10, "BoolText.Text"=w136:string, "BoolText.TextColor"=w129:u32, "BoolText.FontBold"=w135:bool, "BoolText.FontName"=w134:string, "BoolText.FontSize"=w133:u32, "BoolText.Position"=w128:T8)  [unwired: 1 in, 4 out]
        n84 = Subtract(x=w128, y=cluster{"Left":i32, "Top":i32} {"Left"=24, "Top"=36}) -> (x-y=w126:T8)
        n85 = Bundle By Name(cluster=T5 {"False Color"=16777215, "True Color"=16777215, "True Press"=16777215, "False Press"=16777215} ("Multiple Colors"), "False Color"=w129, "True Color"=w129, "True Press"=w129, "False Press"=w129) -> (w130:T5)
        n86 = Bundle By Name(cluster=T2 {"Font:Color"=13140, "Font:Bold?"=TRUE, "Font:Name"="App Font", "Font:Size"=22} ("Boolean Text Format"), "Font:Color"=w129, "Font:Bold?"=w135, "Font:Name"=w134, "Font:Size"=w133) -> (w132:T2)
        n87 = local write "Multiple Colors"(w130) -> ()
        n88 = local write "Image Color"(w129) -> ()
        n89 = local write "Button Size"(w138) -> ()
        n90 = local write "Boolean Text"(w136) -> ()
        n91 = local write "Boolean Text Format"(w132) -> ()
        n92 = local write "Button Text Location"(w126) -> ()
      }
      event User Event {
        w170 = FALSE ("Wait Until Done")
        # "run and reinsert the VI"
        # "abort to make the change"
        n93 = event-data() -> ()  [unwired: 1 in, 1 out]
        n94 = property on="Button Family" class="Ring (strict)"() -> ("RingText.Text"=w152:string)  [unwired: 2 in, 2 out]
        n95 = Unbundle By Name(w147) -> ("subpanel VI path"=w148:path, "Editor Theme"=w149:refnum<class "Material Theme.lvclass">, "subpanel VI ref"=w150:refnum<vi>)
        n96 = case shown="\"(3) Large Button Single Image 40px\", \"(6) Large Button Multi Image 40px\"" w152 {
          tunnel: [path "../_button-editor/add_reaction.png" path "../_button-editor/add_reaction_big.png"] -> w151
          frame Default {
          }
          frame "(3) Large Button Single Image 40px", "(6) Large Button Multi Image 40px" {
          }
        }
        n97 = invoke on="Button Preview" class="SubPnl" method="Remove VI"() -> (error out=w163:errorcluster)  [unwired: 3 in, 2 out]
        n98 = local read "Theme"() -> (w169:u16)
        n99 = invoke class="VI" method="Abort VI"(reference=w150, error in=w163) -> (reference out=w167:refnum<vi>, error out=w171:errorcluster)  [unwired: 1 in, 1 out]
        n100 = call "Get Scheme.vi"("Theme"=w169, "Material Theme in"=w149) -> ("Material-Scheme"=w164:refnum<class "Material-Scheme.lvclass">)  [unwired: 7 in, 2 out]
        n101 = Close Reference(reference=w167, error in (no error)=w171) -> (error out=w168:errorcluster)
        n102 = call <vilib>:"Clear Errors.vi"("error in (no error)"=w168) -> ("error out"=w166:errorcluster)  [unwired: 5 in, 1 out]
        n103 = Current VI's Path() -> (path=w155:path)
        n104 = Build Path(base path=w155, name or relative path=w151) -> (appended path=w154:path)
        n105 = Empty String/Path?(string/path="Button Image") -> (empty?=w157:bool)
        n106 = Select(t=w154, s=w157, f="Button Image") -> (s? t:f=w153:path)
        n107 = call "Scheme.Update Image.vi"("Replace Image"=w153, "error in"=w166, "New Color"="Image Color", "New Control"=w148, "Material-Scheme.lvclass"=w164) -> ("error out"=w165:errorcluster)  [unwired: 5 in, 1 out]
        n108 = Open VI Reference(vi path=w148, error in (no error)=w165) -> (vi reference=w162:refnum<vi>, error out=w161:errorcluster)  [unwired: 4 in]
        n109 = invoke on="Button Preview" class="SubPnl" method="Insert VI"(error in=w161, "VI Ref"=w162) -> (error out=w160:errorcluster)  [unwired: 2 in, 3 out]
        n110 = invoke class="VI" method="Run VI"(reference=w162, error in=w160, "Wait until done"=w170, "Auto Dispose Ref"=w170) -> (reference out=w145:refnum<vi>, error out=w158:errorcluster)  [unwired: 1 in, 3 out]
        n111 = Bundle By Name(cluster=w147, "subpanel VI ref"=w145) -> (w146:refnum<class "TSC Button Editor.lvclass">)
      }
      event User Event {
        w203 = FALSE ("Wait Until Done")
        # "run and reinsert the VI"
        # "abort to make the change"
        n112 = event-data() -> ()  [unwired: 1 in, 1 out]
        n113 = property on="Button Family" class="Ring (strict)"() -> ("RingText.Text"=w181:string)  [unwired: 2 in, 2 out]
        n114 = Unbundle By Name(w176) -> ("subpanel VI path"=w177:path, "Editor Theme"=w178:refnum<class "Material Theme.lvclass">, "subpanel VI ref"=w179:refnum<vi>)
        n115 = case shown="\"(3) Large Button Single Image 40px\", \"(6) Large Button Multi Image 40px\"" w181 {
          tunnel: [path "../_button-editor/add_reaction.png" path "../_button-editor/add_reaction_big.png"] -> w180
          frame Default {
          }
          frame "(3) Large Button Single Image 40px", "(6) Large Button Multi Image 40px" {
          }
        }
        n116 = invoke on="Button Preview" class="SubPnl" method="Remove VI"() -> (error out=w196:errorcluster)  [unwired: 3 in, 2 out]
        n117 = local read "Theme"() -> (w202:u16)
        n118 = invoke class="VI" method="Abort VI"(reference=w179, error in=w196) -> (reference out=w200:refnum<vi>, error out=w204:errorcluster)  [unwired: 1 in, 1 out]
        n119 = call "Get Scheme.vi"("Theme"=w202, "Material Theme in"=w178) -> ("Material-Scheme"=w197:refnum<class "Material-Scheme.lvclass">)  [unwired: 7 in, 2 out]
        n120 = Close Reference(reference=w200, error in (no error)=w204) -> (error out=w201:errorcluster)
        n121 = Cluster To Array(cluster="Multiple Colors") -> (array=w182:u32[])
        n122 = Cluster To Array(cluster="Button Images") -> (array=w184:path[])
        n123 = call <vilib>:"Clear Errors.vi"("error in (no error)"=w201) -> ("error out"=w199:errorcluster)  [unwired: 5 in, 1 out]
        n124 = Current VI's Path() -> (path=w191:path)
        n125 = Build Path(base path=w191, name or relative path=w180) -> (appended path=w190:path)
        n126 = for {
          N: 4 -> [_]
          tunnel: w190 -> [w214]
          tunnel: [w213] -> w189 mode=indexing
          tunnel: w184 -> [w212]
          i -> [w210]
          n127 = Index Array(array=w212, index=w210) -> (element=w211:path)
          n128 = Empty String/Path?(string/path=w211) -> (empty?=w215:bool)
          n129 = Select(t=w214, s=w215, f=w211) -> (s? t:f=w213:path)
        }
        n130 = for {
          N: 4 -> [_]
          tunnel: [w208] -> w186 mode=indexing
          tunnel: w182 -> [w207]
          i -> [w209]
          n131 = Index Array(array=w207, index=w209) -> (element=w208:u32)
        }
        n132 = call "Scheme.Update Image (Multiple).vi"("Replace Image"=w189, "error in"=w199, "New Color"=w186, "New Control"=w177, "Material-Scheme.lvclass"=w197) -> ("error out"=w198:errorcluster)  [unwired: 4 in, 2 out]
        n133 = Open VI Reference(vi path=w177, error in (no error)=w198) -> (vi reference=w195:refnum<vi>, error out=w194:errorcluster)  [unwired: 4 in]
        n134 = invoke on="Button Preview" class="SubPnl" method="Insert VI"(error in=w194, "VI Ref"=w195) -> (error out=w193:errorcluster)  [unwired: 2 in, 3 out]
        n135 = invoke class="VI" method="Run VI"(reference=w195, error in=w193, "Wait until done"=w203, "Auto Dispose Ref"=w203) -> (reference out=w174:refnum<vi>, error out=w192:errorcluster)  [unwired: 1 in, 3 out]
        n136 = Bundle By Name(cluster=w176, "subpanel VI ref"=w174) -> (w175:refnum<class "TSC Button Editor.lvclass">)
      }
      event "update colors", "Boolean Colors": Value Change {
        w223 = refnum<vi> refnum  # Boolean
        n137 = event-data() -> ()  [unwired: 1 in, 1 out]
        n138 = Unbundle By Name(w219) -> ("subpanel VI ref"=w217:refnum<vi>)
        n139 = Unbundle By Name("Boolean Colors") -> ("false color"=w231:cluster{"border":u32, "fill":u32}, "true color"=w230:cluster{"border":u32, "fill":u32}, "click true color"=w225:cluster{"border":u32, "fill":u32}, "click false color"=w226:cluster{"border":u32, "fill":u32}, "hover false color"=w229:cluster{"border":u32, "fill":u32}, "hover true color"=w228:cluster{"border":u32, "fill":u32})
        n140 = property class="VI"(reference=w217) -> ("Panel"=w236:refnum<vi>)  [unwired: 1 in, 2 out]
        n141 = property class="Pnl"(reference=w236) -> (error out=w234:errorcluster, "Controls[]"=w221:refnum<vi>[])  [unwired: 1 in, 1 out]
        n142 = Build Array(w231, w230, w225, w226, w229, w228) -> (w227:cluster{"border":u32, "fill":u32}[])
        n143 = Index Array(array=w221) -> (element=w220:refnum<vi>)  [unwired: 1 in]
        n144 = To More Specific Class(target class=w223, reference=w220, error in=w234) -> (specific class reference=w224:refnum<vi>, error out=w222:errorcluster)
        n145 = property class="Bool"(reference=w224, error in=w222, "Colors [4]"=w227) -> (error out=w235:errorcluster)  [unwired: 1 out]
        n146 = invoke class="VI" method="Save.Instrument"(reference=w217, error in=w235) -> (reference out=w216:refnum<vi>, error out=w233:errorcluster)  [unwired: 4 in, 4 out]
        n147 = Bundle By Name(cluster=w219, "subpanel VI ref"=w216) -> (w218:refnum<class "TSC Button Editor.lvclass">)
      }
      event "Boolean Text": Value Change {
        w243 = refnum<vi> refnum  # Boolean
        n148 = event-data() -> ()  [unwired: 1 in, 1 out]
        n149 = Unbundle By Name(w238) -> ("subpanel VI ref"=w240:refnum<vi>)
        n150 = property class="VI"(reference=w240) -> ("Panel"=w250:refnum<vi>)  [unwired: 1 in, 2 out]
        n151 = property class="Pnl"(reference=w250) -> (error out=w247:errorcluster, "Controls[]"=w249:refnum<vi>[])  [unwired: 1 in, 1 out]
        n152 = Index Array(array=w249) -> (element=w241:refnum<vi>)  [unwired: 1 in]
        n153 = To More Specific Class(target class=w243, reference=w241, error in=w247) -> (specific class reference=w244:refnum<vi>, error out=w242:errorcluster)
        n154 = property class="Bool"(reference=w244, error in=w242, "BoolText.Text"="Boolean Text") -> (error out=w248:errorcluster)  [unwired: 1 out]
        n155 = invoke class="VI" method="Save.Instrument"(reference=w240, error in=w248) -> (reference out=w239:refnum<vi>, error out=w245:errorcluster)  [unwired: 4 in, 4 out]
        n156 = Bundle By Name(cluster=w238, "subpanel VI ref"=w239) -> (w237:refnum<class "TSC Button Editor.lvclass">)
      }
      event "Button Size", "update button size": Value Change {
        w260 = refnum<vi> refnum  # Boolean
        n157 = event-data() -> ()  [unwired: 1 in, 1 out]
        n158 = Unbundle By Name(w252) -> ("subpanel VI ref"=w254:refnum<vi>)
        n159 = property class="VI"(reference=w254) -> ("Panel"=w263:refnum<vi>)  [unwired: 1 in, 2 out]
        n160 = property class="Pnl"(reference=w263) -> ("Controls[]"=w259:refnum<vi>[])  [unwired: 1 in, 2 out]
        n161 = Index Array(array=w259) -> (element=w262:refnum<vi>)  [unwired: 1 in]
        n162 = To More Specific Class(target class=w260, reference=w262) -> (specific class reference=w261:refnum<vi>, error out=w257:errorcluster)  [unwired: 1 in]
        n163 = property class="Bool"(reference=w261, error in=w257, "Button Size"="Button Size") -> (error out=w256:errorcluster)  [unwired: 1 out]
        n164 = invoke class="VI" method="Save.Instrument"(reference=w254, error in=w256) -> (reference out=w253:refnum<vi>, error out=w255:errorcluster)  [unwired: 4 in, 4 out]
        n165 = Bundle By Name(cluster=w252, "subpanel VI ref"=w253) -> (w251:refnum<class "TSC Button Editor.lvclass">)
      }
      event "update button text location", "Button Text Location": Value Change {
        w274 = refnum<vi> refnum  # Boolean
        n166 = event-data() -> ()  [unwired: 1 in, 1 out]
        n167 = Unbundle By Name(w267) -> ("subpanel VI ref"=w268:refnum<vi>)
        n168 = property class="VI"(reference=w268) -> ("Panel"=w277:refnum<vi>)  [unwired: 1 in, 2 out]
        n169 = property class="Pnl"(reference=w277) -> ("Controls[]"=w273:refnum<vi>[])  [unwired: 1 in, 2 out]
        n170 = Index Array(array=w273) -> (element=w276:refnum<vi>)  [unwired: 1 in]
        n171 = To More Specific Class(target class=w274, reference=w276) -> (specific class reference=w275:refnum<vi>)  [unwired: 1 in, 1 out]
        n172 = Add(x="Button Text Location", y=cluster{"Left":i32, "Top":i32} {"Left"=24, "Top"=36}) -> (x+y=w271:cluster{"Left":i32, "Top":i32})
        n173 = property class="Bool"(reference=w275, "BoolText.Position"=w271) -> (error out=w265:errorcluster)  [unwired: 1 in, 1 out]
        n174 = invoke class="VI" method="Save.Instrument"(reference=w268, error in=w265) -> (reference out=w269:refnum<vi>, error out=w264:errorcluster)  [unwired: 4 in, 4 out]
        n175 = Bundle By Name(cluster=w267, "subpanel VI ref"=w269) -> (w266:refnum<class "TSC Button Editor.lvclass">)
      }
      event "Lock Text in Center?": Value Change {
        w289 = refnum<vi> refnum  # Boolean
        n176 = event-data() -> ()  [unwired: 1 in, 1 out]
        n177 = Unbundle By Name(w279) -> ("subpanel VI ref"=w278:refnum<vi>)
        n178 = property class="VI"(reference=w278) -> ("Panel"=w292:refnum<vi>)  [unwired: 1 in, 2 out]
        n179 = property class="Pnl"(reference=w292) -> ("Controls[]"=w288:refnum<vi>[])  [unwired: 1 in, 2 out]
        n180 = Index Array(array=w288) -> (element=w291:refnum<vi>)  [unwired: 1 in]
        n181 = To More Specific Class(target class=w289, reference=w291) -> (specific class reference=w290:refnum<vi>)  [unwired: 1 in, 1 out]
        n182 = property class="Bool"(reference=w290, "LockBoolText"="Lock Text in Center?") -> (error out=w282:errorcluster, "BoolText.Position"=w284:T8)  [unwired: 1 in, 1 out]
        n183 = Subtract(x=w284, y=cluster{"Left":i32, "Top":i32} {"Left"=24, "Top"=36}) -> (x-y=w286:T8)
        n184 = local write "Button Text Location"(w286) -> ()
        n185 = invoke class="VI" method="Save.Instrument"(reference=w278, error in=w282) -> (reference out=w283:refnum<vi>, error out=w281:errorcluster)  [unwired: 4 in, 4 out]
        n186 = Bundle By Name(cluster=w279, "subpanel VI ref"=w283) -> (w280:refnum<class "TSC Button Editor.lvclass">)
      }
      event "Boolean Text Format", "update text format": Value Change {
        w302 = refnum<vi> refnum  # Boolean
        n187 = event-data() -> ()  [unwired: 1 in, 1 out]
        n188 = Unbundle By Name(w294) -> ("subpanel VI ref"=w293:refnum<vi>)
        n189 = property class="VI"(reference=w293) -> ("Panel"=w310:refnum<vi>)  [unwired: 1 in, 2 out]
        n190 = Unbundle By Name("Boolean Text Format") -> ("Font:Color"=w307:u32, "Font:Bold?"=w306:bool, "Font:Name"=w305:string, "Font:Size"=w304:u32)
        n191 = property class="Pnl"(reference=w310) -> (error out=w309:errorcluster, "Controls[]"=w300:refnum<vi>[])  [unwired: 1 in, 1 out]
        n192 = Index Array(array=w300) -> (element=w299:refnum<vi>)  [unwired: 1 in]
        n193 = To More Specific Class(target class=w302, reference=w299, error in=w309) -> (specific class reference=w303:refnum<vi>, error out=w301:errorcluster)
        n194 = property class="Bool"(reference=w303, error in=w301, "BoolText.FontColor"=w307, "BoolText.TextColor"=w307, "BoolText.FontBold"=w306, "BoolText.FontName"=w305, "BoolText.FontSize"=w304) -> (error out=w297:errorcluster)  [unwired: 1 out]
        n195 = invoke class="VI" method="Save.Instrument"(reference=w293, error in=w297) -> (reference out=w298:refnum<vi>, error out=w296:errorcluster)  [unwired: 4 in, 4 out]
        n196 = Bundle By Name(cluster=w294, "subpanel VI ref"=w298) -> (w295:refnum<class "TSC Button Editor.lvclass">)
      }
      event "Save": Value Change {
        n197 = event-data() -> ()  [unwired: 1 in, 1 out]
        n198 = Unbundle By Name(w313) -> ("subpanel VI ref"=w312:refnum<vi>)
        n199 = call "File Dialog"("pattern (all files)"="*.ctl" ("pattern label")) -> ("selected path"=w315:path, "error out"=w316:errorcluster)  [unwired: 11 in, 2 out]
        n200 = property class="VI"(reference=w312) -> ("Panel"=w320:refnum<vi>)  [unwired: 1 in, 2 out]
        n201 = property class="Pnl"(reference=w320) -> ("Controls[]"=w319:refnum<vi>[])  [unwired: 1 in, 2 out]
        n202 = Index Array(array=w319) -> (element=w318:refnum<vi>)  [unwired: 1 in]
        n203 = case shown="No Error" w316 {
          selector: w316 -> [w332 w341 _]
          tunnel: w318 -> [w337 _ _]
          tunnel: [w334 w341 _] -> w317
          tunnel: w315 -> [w331 _ _]
          tunnel: "Save For:" -> [w321 _ _]
          frame No Error {
            w326 = TRUE  # Is Persistent?
            # "save as a .ctl file with the tag data applied for the control-level"
            n204 = New VI(8:w332, 9:T9."Control VI" ("vi type (standard vi)")) -> (0:w339:errorcluster, 3:w338:refnum<vi>)  [unwired: 5 in]
            n205 = invoke class="VI" method="Create from Reference"(reference=w338, error in=w339, "Source Object Ref"=w337) -> (reference out=w328:refnum<vi>, error out=w336:errorcluster, "New Object Ref"=w330:refnum<vi>)  [unwired: 4 in, 4 out]
            n206 = property on="Color Level" class="Ring (strict)"() -> ("RingText.Text"=w322:string)  [unwired: 2 in, 2 out]
            n207 = property class="Ctl"(reference=w330, error in=w336, "Position"=T8 {"Left"=24, "Top"=18}) -> (reference out=w324:refnum<vi>, error out=w325:errorcluster)
            n208 = invoke class="Ctl" method="Tag.Set Tag"(reference=w324, error in=w325, "TagName"="control-level" ("Tag Name"), "Value"=w322, "isPersistent"=w326) -> (error out=w323:errorcluster)  [unwired: 2 in, 6 out]
            n209 = invoke class="VI" method="Save.For Previous"(reference=w328, error in=w323, "Path to saved file"=w331, "Oldest compatible target version"=w321) -> (reference out=w333:refnum<vi>, error out=w335:errorcluster)  [unwired: 2 in, 4 out]
            n210 = Close Reference(reference=w333, error in (no error)=w335) -> (error out=w334:errorcluster)
          }
          frame Default {
          }
          frame Error {
          }
        }
      }
      event Menu Selection (User) {
        n211 = event-data() -> ("ItemTag"=w344:string)  [unwired: 1 in]
        n212 = Unbundle By Name(w343) -> ("subpanel VI ref"=w342:refnum<vi>)
        n213 = case shown="\"save\"" w344 {
          tunnel: w342 -> [_ w353]
          tunnel: [_ w350] -> w345
          frame Default {
          }
          frame "save" {
            # "Ctrl+S menu shortcut"
            n214 = call "File Dialog3"("pattern (all files)"="*.ctl" ("pattern label")) -> ("selected path"=w348:path, "error out"=w349:errorcluster)  [unwired: 11 in, 2 out]
            n215 = property class="VI"(reference=w353) -> ("Panel"=w354:refnum<vi>)  [unwired: 1 in, 2 out]
            n216 = property class="Pnl"(reference=w354) -> ("Controls[]"=w352:refnum<vi>[])  [unwired: 1 in, 2 out]
            n217 = Index Array(array=w352) -> (element=w351:refnum<vi>)  [unwired: 1 in]
            n218 = local read "Save For:"() -> (w346:string)
            n219 = case shown="No Error" w349 {
              selector: w349 -> [w366 w375 _]
              tunnel: w351 -> [w371 _ _]
              tunnel: [w368 w375 _] -> w350
              tunnel: w348 -> [w365 _ _]
              tunnel: w346 -> [w355 _ _]
              frame No Error {
                n220 = New VI(8:w366, 9:T9."Control VI" ("vi type (standard vi)")) -> (0:w373:errorcluster, 3:w372:refnum<vi>)  [unwired: 5 in]
                n221 = invoke class="VI" method="Create from Reference"(reference=w372, error in=w373, "Source Object Ref"=w371) -> (reference out=w362:refnum<vi>, error out=w370:errorcluster, "New Object Ref"=w364:refnum<vi>)  [unwired: 4 in, 4 out]
                n222 = property on="Color Level" class="Ring (strict)"() -> ("RingText.Text"=w361:string)  [unwired: 2 in, 2 out]
                n223 = property class="Ctl"(reference=w364, error in=w370, "Position"=T8 {"Left"=24, "Top"=18}) -> (reference out=w357:refnum<vi>, error out=w358:errorcluster)
                n224 = invoke class="Ctl" method="Tag.Set Tag"(reference=w357, error in=w358, "TagName"="control-level" ("Tag Name"), "Value"=w361, "isPersistent"=TRUE ("Is Persistent?")) -> (error out=w356:errorcluster)  [unwired: 2 in, 6 out]
                n225 = invoke class="VI" method="Save.For Previous"(reference=w362, error in=w356, "Path to saved file"=w365, "Oldest compatible target version"=w355) -> (reference out=w367:refnum<vi>, error out=w369:errorcluster)  [unwired: 2 in, 4 out]
                n226 = Close Reference(reference=w367, error in (no error)=w369) -> (error out=w368:errorcluster)
              }
              frame Default {
              }
              frame Error {
              }
            }
          }
        }
      }
      event "Button Type": Value Change {
        w402 = FALSE ("Wait Until Done")
        # "rerun and reinsert VI with new control"
        # "open the selected ctl and replace old one"
        # "abort and remove temporarily"
        n227 = event-data() -> ()  [unwired: 1 in, 1 out]
        n228 = Unbundle By Name(w380) -> ("subpanel VI path"=w381:path, "subpanel VI ref"=w377:refnum<vi>, "control top level"=w376:path)
        n229 = Unbundle By Name(w390) -> ("update colors"=w389:refnum<user-event>)
        n230 = invoke class="VI" method="Abort VI"(reference=w377) -> (error out=w395:errorcluster)  [unwired: 2 in, 2 out]
        n231 = property on="Button Family" class="Ring (strict)"() -> ("RingText.Text"=w385:string)  [unwired: 2 in, 2 out]
        n232 = Generate User Event(user event=w389, event data cluster=variant ("event data")) -> ()  [unwired: 2 in, 2 out]
        n233 = invoke on="Button Preview" class="SubPnl" method="Remove VI"(error in=w395) -> (error out=w394:errorcluster)  [unwired: 2 in, 2 out]
        n234 = Build Path(base path=w376, name or relative path=w385) -> (appended path=w386:path)
        n235 = call <vilib>:"Clear Errors.vi"("error in (no error)"=w394) -> ("error out"=w393:errorcluster)  [unwired: 5 in, 1 out]
        n236 = property class="VI"(reference=w377, error in=w393) -> (reference out=w391:refnum<vi>, error out=w398:errorcluster, "Panel"=w412:refnum<vi>)
        n237 = List Folder(path=w386, pattern="*.ctl") -> (path out=w408:path, filenames=w409:string[])  [unwired: 2 in, 2 out]
        n238 = property class="Pnl"(reference=w412, error in=w398) -> (error out=w397:errorcluster, "Controls[]"=w411:refnum<vi>[])  [unwired: 1 out]
        n239 = Index Array "Index Array"(array=w409, index="Button Type") -> (element=w407:string)
        n240 = Index Array(array=w411) -> (element=w406:refnum<vi>)  [unwired: 1 in]
        n241 = Build Path(base path=w408, name or relative path=w407) -> (appended path=w387:path)
        n242 = invoke class="Ctl" method="Replace No Attrib"(reference=w406, error in=w397, "Param 1"=w387) -> (error out=w399:errorcluster, "RepNoAttrib"=w382:refnum<vi>)  [unwired: 3 in, 4 out]
        n243 = property class="GObj"(reference=w382, error in=w399, "Position"=T8 {"Left"=0, "Top"=0}) -> (error out=w384:errorcluster)  [unwired: 1 out]
        n244 = invoke class="VI" method="Save.Instrument"(reference=w391, error in=w384) -> (error out=w392:errorcluster)  [unwired: 4 in, 5 out]
        n245 = Close Reference(reference=w391, error in (no error)=w392) -> (error out=w400:errorcluster)
        n246 = Open VI Reference(vi path=w381, error in (no error)=w400) -> (vi reference=w403:refnum<vi>, error out=w404:errorcluster)  [unwired: 4 in]
        n247 = invoke class="VI" method="Run VI"(reference=w403, error in=w404, "Wait until done"=w402, "Auto Dispose Ref"=w402) -> (reference out=w378:refnum<vi>, error out=w396:errorcluster)  [unwired: 1 in, 3 out]
        n248 = Bundle By Name(cluster=w380, "subpanel VI ref"=w378) -> (w379:refnum<class "TSC Button Editor.lvclass">)
        n249 = invoke on="Button Preview" class="SubPnl" method="Insert VI"(error in=w396, "VI Ref"=w378) -> (error out=w401:errorcluster)  [unwired: 2 in, 3 out]
      }
      event "Button Family": Value Change {
        w417 = u16 0 items=[""] ("Button Type")
        n250 = event-data() -> ()  [unwired: 1 in, 1 out]
        n251 = property on="Button Family" class="Ring (strict)"() -> ("RingText.Text"=w415:string)  [unwired: 2 in, 2 out]
        n252 = Unbundle By Name(w414) -> ("control top level"=w413:path)
        n253 = case shown="\"(2) Small Button Text Only\", \"(4) Large Button Text Only\"" w415 {
          tunnel: [TRUE FALSE FALSE] -> w421
          tunnel: [FALSE TRUE FALSE] -> w420
          frame Default {
          }
          frame "(5) Small Button Multi Image 24px", "(6) Large Button Multi Image 40px" {
          }
          frame "(2) Small Button Text Only", "(4) Large Button Text Only" {
          }
        }
        n254 = property on="Button Image" class="Path"("Visible"=w421) -> ()  [unwired: 2 in, 2 out]
        n255 = property on="Button Images" class="Clust (strict)"("Visible"=w420) -> ()  [unwired: 2 in, 2 out]
        n256 = property on="Image Color" class="ColBox"("Visible"=w421) -> ()  [unwired: 2 in, 2 out]
        n257 = property on="Multiple Colors" class="Clust (strict)"("Visible"=w420) -> ()  [unwired: 2 in, 2 out]
        n258 = Build Path(base path=w413, name or relative path=w415) -> (appended path=w419:path)
        n259 = List Folder(path=w419, pattern="*.ctl") -> (filenames=w416:string[])  [unwired: 2 in, 3 out]
        n260 = property on="Button Type" class="Ring (strict)"("Strings []"=w416, "Val(Sgnl)"=w417) -> ()  [unwired: 2 in, 2 out]
      }
      event "Open": Value Change {
        n261 = event-data() -> ()  [unwired: 1 in, 1 out]
        n262 = call "File Dialog2"("pattern label"="*.ctl") -> ("selected path"=w430:path, "error out"=w432:errorcluster)  [unwired: 11 in, 2 out]
        n263 = case shown="No Error" w432 {
          selector: w432 -> [_ w516]
          tunnel: [w453 w515] -> w431
          tunnel: w430 -> [w458 _]
          tunnel: w429 -> [w446 w514]
          tunnel: [w444 w514] -> w428
          frame No Error {
            w455 = FALSE ("Wait Until Done")
            w486 = refnum<vi> refnum  # Boolean
            # "icon-images"
            # "#update \nNeeds:\n-pull out the meta-data for the button type\n-how the heck do i figure out the theme file it was saved with?? - add other tag?? hmmm........\n-need color of image also"
            n264 = Unbundle By Name(w446) -> ("subpanel VI path"=w448:path, "subpanel VI ref"=w449:refnum<vi>)
            n265 = invoke on="Button Preview" class="SubPnl" method="Remove VI"() -> (error out=w457:errorcluster)  [unwired: 3 in, 2 out]
            n266 = invoke class="VI" method="Abort VI"(reference=w449, error in=w457) -> (reference out=w463:refnum<vi>, error out=w469:errorcluster)  [unwired: 1 in, 1 out]
            n267 = Close Reference(reference=w463, error in (no error)=w469) -> (error out=w467:errorcluster)
            n268 = call <vilib>:"Clear Errors.vi"("error in (no error)"=w467) -> ("error out"=w466:errorcluster)  [unwired: 5 in, 1 out]
            n269 = Open VI Reference(vi path=w458, error in (no error)=w466) -> (vi reference=w464:refnum<vi>, error out=w465:errorcluster)  [unwired: 4 in]
            n270 = property class="VI"(reference=w464, error in=w465) -> (reference out=w459:refnum<vi>, error out=w485:errorcluster, "Panel"=w487:refnum<vi>)
            n271 = property class="Pnl"(reference=w487, error in=w485) -> (error out=w484:errorcluster, "Controls[]"=w490:refnum<vi>[])  [unwired: 1 out]
            n272 = Index Array(array=w490) -> (element=w488:refnum<vi>)  [unwired: 1 in]
            n273 = To More Specific Class(target class=w486, reference=w488, error in=w484) -> (specific class reference=w489:refnum<vi>, error out=w468:errorcluster)
            n274 = property class="Bool" props=["BoolText", "Position", "Label", "Height", "Button Size", "BoolText", "Text", "BoolText", "TextColor", "BoolText", "FontBold", "BoolText", "FontName", "BoolText", "FontSize", "Colors [4]", "LockBoolText"](reference=w489, error in=w468) -> (error out=w462:errorcluster, "BoolText.Position"=w440:T8, "Button Size"=w483:T10, "BoolText.Text"=w482:string, "BoolText.TextColor"=w481:u32, "BoolText.FontBold"=w480:bool, "BoolText.FontName"=w479:string, "BoolText.FontSize"=w478:u32, "Colors [4]"=w474:cluster{u32, u32}[], "LockBoolText"=w443:bool)  [unwired: 2 out]
            n275 = Close Reference(reference=w459, error in (no error)=w462) -> (error out=w460:errorcluster)
            n276 = Index Array(array=w474) -> (element #1=w473:cluster{u32, u32}, element #2=w472:cluster{u32, u32}, element #3=w471:cluster{u32, u32}, element #4=w470:cluster{u32, u32})  [unwired: 6 in, 2 out]
            n277 = property on="Color Level" class="Ring (strict)"() -> ("Strings []"=w439:string[])  [unwired: 2 in, 2 out]
            n278 = Open VI Reference(vi path=w448, error in (no error)=w460) -> (vi reference=w451:refnum<vi>, error out=w461:errorcluster)  [unwired: 4 in]
            n279 = local read "Boolean Colors"() -> (w447:T1)
            n280 = Bundle By Name(cluster=w447, "false color"=w473, "true color"=w472, "click true color"=w471, "click false color"=w470) -> (w475:T1)
            n281 = call "Update Custom UI for Button.vi"("error in"=w461, "selected path"=w458, "vi reference"=w451) -> ("error out"=w454:errorcluster, "appended path"=w452:path, "vi reference out"=w450:refnum<vi>, "icon-images"=w436:string, "control-level"=w437:string)  [unwired: 4 in]
            n282 = Search 1D Array(1D array=w439, element=w437) -> (index of element=w438:i32)  [unwired: 1 in]
            n283 = Subtract(x=w440, y=cluster{"Left":i32, "Top":i32} {"Left"=24, "Top"=36}) -> (x-y=w442:T8)
            n284 = Bundle By Name(cluster=T2 {"Font:Color"=3563918, "Font:Bold?"=TRUE, "Font:Name"="App Font", "Font:Size"=22} ("Boolean Text Format"), "Font:Color"=w481, "Font:Bold?"=w480, "Font:Name"=w479, "Font:Size"=w478) -> (w477:T2)
            n285 = invoke on="Button Preview" class="SubPnl" method="Insert VI"(error in=w454, "VI Ref"=w450) -> (error out=w456:errorcluster)  [unwired: 2 in, 3 out]
            n286 = property on="Color Level" class="Ring (strict)"("Value"=w438) -> ()  [unwired: 2 in, 2 out]
            n287 = invoke class="VI" method="Run VI"(reference=w450, error in=w456, "Wait until done"=w455, "Auto Dispose Ref"=w455) -> (reference out=w445:refnum<vi>, error out=w453:errorcluster)  [unwired: 1 in, 3 out]
            n288 = local write "Button Text Location"(w442) -> ()
            n289 = local write "Button Size"(w483) -> ()
            n290 = local write "Boolean Text"(w482) -> ()
            n291 = local write "Boolean Text Format"(w477) -> ()
            n292 = local write "Boolean Colors"(w475) -> ()
            n293 = local write "Lock Text in Center?"(w443) -> ()
            n294 = flat-sequence {
              tunnel: w452 -> [w494]
              tunnel: w453 -> [_]
              tunnel: w436 -> [w493]
              tunnel: [w492] -> w435
              tunnel: [w491] -> w434
              frame #0 {
                n295 = case shown="\"four-panel\"" w493 {
                  tunnel: w494 -> [w498 w509]
                  tunnel: [TRUE FALSE] -> w492
                  tunnel: [FALSE TRUE] -> w491
                  frame "single", Default {
                    n296 = call "Read Image on Button.vi"("File with Button"=w498) -> ("png file out"=w497:path)  [unwired: 9 in, 1 out]
                    n297 = local write "Button Image"(w497) -> ()
                  }
                  frame "four-panel" {
                    n298 = for {
                      N: 4 -> [_]
                      tunnel: w509 -> [w513]
                      tunnel: [w511] -> w508 mode=indexing
                      i -> [w512]
                      n299 = call "Read Image on Button.vi"("Append Name?"=TRUE, "image item"=w512, "File with Button"=w513) -> ("png file out"=w511:path)  [unwired: 7 in, 1 out]
                    }
                    n300 = Index Array(array=w508) -> (element #1=w506:path, element #2=w504:path, element #3=w503:path, element #4=w502:path)  [unwired: 4 in]
                    n301 = Bundle(cluster=T4 {"False Image"=path "", "True Image"=path "", "True Press"=path "", "False Press"=path ""} ("Button Images"), "False Image"=w506, "True Image"=w504, "True Press"=w503, "False Press"=w502) -> (w505:T4)
                    n302 = local write "Button Images"(w505) -> ()
                  }
                }
              }
            }
            n303 = property on="Button Image" class="Path"("Visible"=w435) -> ()  [unwired: 2 in, 2 out]
            n304 = property on="Button Images" class="Clust (strict)"("Visible"=w434) -> ()  [unwired: 2 in, 2 out]
            n305 = Bundle By Name(cluster=w446, "subpanel VI ref"=w445) -> (w444:refnum<class "TSC Button Editor.lvclass">)
            n306 = property on="Image Color" class="ColBox"("Visible"=w435) -> ()  [unwired: 2 in, 2 out]
            n307 = property on="Multiple Colors" class="Clust (strict)"("Visible"=w434) -> ()  [unwired: 2 in, 2 out]
          }
          frame Error {
            n308 = Unbundle By Name(w516) -> ("code"=w517:i32)
            n309 = case shown="43" w517 {
              tunnel: w516 -> [w518 _]
              tunnel: [w518 _] -> w515
              frame Default {
              }
              frame 43 {
              }
            }
          }
        }
      }
      event "edit": Value Change {
        n310 = event-data() -> ()  [unwired: 1 in, 1 out]
        n311 = call "File Dialog4"() -> ("selected path"=w520:path, "error out"=w523:errorcluster)  [unwired: 12 in, 2 out]
        n312 = case shown="No Error" w523 {
          selector: w523 -> [w530 w532 _]
          tunnel: [w527 w532 errorcluster {"status"=FALSE, "code"=0, "source"=""} ("error IO")] -> w522
          tunnel: w521 -> [w529 w531 w533]
          tunnel: w520 -> [w526 _ _]
          tunnel: [w525 w531 w533] -> w519
          frame No Error {
            n313 = call "Change Image Directory.vi"("error in"=w530, "Image Dir"=w526, "TSC Button Editor in"=w529) -> ("error out"=w527:errorcluster, "TSC Button Editor out"=w525:refnum<class "TSC Button Editor.lvclass">, "Images"=w528:T3)  [unwired: 6 in]
            n314 = Unbundle By Name(w525) -> ("image directory"=w524:path)
            n315 = local write "Images"(w528) -> ()
            n316 = local write "images directory"(w524) -> ()
          }
          frame Default {
          }
          frame Error {
          }
        }
      }
      event "Filter": Value Change {
        n317 = event-data() -> ("NewVal"=w544:string)  [unwired: 1 in]
        n318 = To Lower Case(string=w544) -> (all lower case string=w549:string)
        n319 = Spreadsheet String To Array(delimiter (Tab)=" ", format string="%s", spreadsheet string=w549, array type (2D Dbl)=string[] []) -> (array=w545:string[])
        n320 = for {
          tunnel: w545 -> [w567] mode=indexing
          tunnel: [w567] -> w542 mode=indexing if=w565
          # "grab all the letters"
          n321 = Empty String/Path?(string/path=w567) -> (empty?=w566:bool)
          n322 = Not(x=w566) -> (.not. x?=w565:bool)
        }
        n323 = Unbundle By Name(w543) -> ("Images"=w535:T6, "Image Names"=w539:string[])
        n324 = for {
          tunnel: w539 -> [w559] mode=indexing
          tunnel: w542 -> [w560]
          tunnel: [w557] -> w541 mode=indexing if=w555
          i -> [w557]
          # "find what names match the filter"
          n325 = To Lower Case(string=w559) -> (all lower case string=w558:string)
          n326 = for {
            tunnel: w560 -> [w564] mode=indexing
            tunnel: w558 -> [w563]
            tunnel: [w561] -> w556
            stop <- w561 stop-if-true
            n327 = Search/Split String(string=w563, search string/char (-)=w564) -> (offset of match=w562:i32)  [unwired: 3 out]
            n328 = Less Than 0?(x=w562) -> (x < 0?=w561:bool)
          }
          n329 = Not(x=w556) -> (.not. x?=w555:bool)
        }
        n330 = for {
          tunnel: w541 -> [w551] mode=indexing
          tunnel: [w554] -> w537 mode=indexing
          tunnel: w535 -> [w553]
          tunnel: w539 -> [w552]
          tunnel: [w550] -> w538 mode=indexing
          # "remove the array items"
          n331 = Delete From Array "Delete From Array"(array=w553, index=w551) -> (deleted portion=w554:T11)  [unwired: 1 in, 1 out]
          n332 = Delete From Array "Delete From Array"(array=w552, index=w551) -> (deleted portion=w550:string)  [unwired: 1 in, 1 out]
        }
        n333 = call "Sort Image Table.vi"("Images in"=w537) -> ("Images out"=w536:T3)  [unwired: 2 in]
        n334 = local write "Images"(w536) -> ()
        n335 = Bundle By Name(cluster=w543, "Filtered Image Names"=w538) -> (w540:refnum<class "TSC Button Editor.lvclass">)
      }
      event "Images": Mouse Down {
        n336 = event-data() -> ("CtlRef"=w570:refnum<vi>, "Coords"=w569:T12)  [unwired: 1 in]
        n337 = call "Array Point to RowCol.vi"("Mouse Coords"=w569, "Array Ref"=w570) -> ("Clicked Index"=w572:i32[])  [unwired: 6 in, 3 out]
        n338 = local read "Images"() -> (w568:T3)
        n339 = Index Array(array=w572) -> (element #1=w573:i32, element #2=w574:i32)  [unwired: 2 in]
        n340 = Index Array "Index Array"(array=w568, index (row)=w573, index (col)=w574) -> (element=w575:T11)
        n341 = Unbundle By Name(w575) -> ("path"=w577:path)
        n342 = Bundle By Name(cluster=cluster{"data name":string, "drag data":variant} {"data name"="array.data", "drag data"=variant}, "drag data"=w577) -> (w576:cluster{"data name":string, "drag data":variant})
        n343 = Build Array(w576) -> (w578:T13)
        n344 = invoke on="Images" class="Arr (strict)" method="Start Drag"("Data"=w578) -> ()  [unwired: 4 in, 5 out]
      }
      event "Button Image", "Button Images.False Image", "Button Images.True Image", "Button Images.True Press", "Button Images.False Press": Drag Enter {
        n345 = event-data() -> ("Available Data Names"=w588:string[])  [unwired: 1 in]
        n346 = Search 1D Array(1D array=w588, element="array.data") -> (index of element=w587:i32)  [unwired: 1 in]
        n347 = Greater Or Equal To 0?(x=w587) -> (x >= 0?=w586:bool)
        n348 = Get Drag Drop Data(8:path "", 9:"array.data" ("data name")) -> (3:w583:path)  [unwired: 1 in, 1 out]
        n349 = Empty String/Path?(string/path=w583) -> (empty?=w581:bool)
        n350 = Not(x=w581) -> (.not. x?=w580:bool)
        n351 = And(x=w586, y=w580) -> (x .and. y?=w582:bool)
        n352 = event-data("Accepted?"=w582) -> ()  [unwired: 1 in, 1 out]
      }
      event "Button Image", "Button Images.False Image", "Button Images.True Image", "Button Images.True Press", "Button Images.False Press": Drop {
        n353 = event-data() -> ("Available Data Names"=w594:string[], "CtlRef"=w591:refnum<vi>)  [unwired: 1 in]
        n354 = Search 1D Array(1D array=w594, element="array.data") -> (index of element=w596:i32)  [unwired: 1 in]
        n355 = Greater Or Equal To 0?(x=w596) -> (x >= 0?=w593:bool)
        n356 = case shown="True" w593 {
          tunnel: [_ w599] -> w592
          tunnel: w591 -> [_ w598]
          frame False {
          }
          frame True {
            n357 = Get Drag Drop Data(8:path "", 9:"array.data" ("data name")) -> (0:w601:errorcluster, 3:w600:path)  [unwired: 1 in]
            n358 = case shown="No Error" w601 {
              tunnel: w600 -> [w606 _]
              tunnel: [w605 _] -> w599
              tunnel: w598 -> [w604 _]
              frame No Error {
                n359 = Empty String/Path?(string/path=w606) -> (empty?=w607:bool)
                n360 = case shown="False" w607 {
                  tunnel: w606 -> [w610 _]
                  tunnel: [TRUE _] -> w605
                  tunnel: w604 -> [w608 _]
                  frame False {
                    n361 = property on="Property Node" class="Path"(reference=w608, "Val(Sgnl)"=w610) -> ()  [unwired: 1 in, 2 out]
                  }
                  frame True {
                  }
                }
              }
              frame Error {
              }
            }
          }
        }
        n362 = event-data("Accepted?"=w592) -> ()  [unwired: 1 in, 1 out]
      }
    }
    "error out" <- w36
    n363 = call <vilib>:"Simple Error Handler.vi"("error in (no error)"=w36) -> ()  [unwired: 4 in, 5 out]
  }
  n364 = call "User Event Close.vi"("Event Registration Refnum"=w28, "user events"=w27) -> ()  [unwired: 9 in, 1 out]
  n365 = Unbundle By Name(w3) -> ("subpanel VI ref"=w11:refnum<vi>)
  n366 = call "Save Editor Data.vi"("TSC Button Editor"=w3) -> ()  [unwired: 10 in, 1 out]
  n367 = flat-sequence {
    tunnel: w3 -> [_]
    frame #0 {
      n368 = control-ref of="This VI"() -> (w611:refnum<vi>)
      n369 = invoke class="VI" method="FP.Close"(reference=w611) -> ()  [unwired: 2 in, 3 out]
    }
  }
  n370 = invoke class="VI" method="Abort VI"(reference=w11) -> (reference out=w33:refnum<vi>, error out=w32:errorcluster)  [unwired: 2 in, 1 out]
  n371 = Close Reference(reference=w33, error in (no error)=w32) -> ()  [unwired: 1 out]
